vi "Retrieve and visulize data_SE.vi"(11 "Field/Temperature":i32(slide) min=0 max=36 step=1 scale=-1.1..1.0) -> (1 "slowest":dbl=-2499.957 format="%#_6p")   [LabVIEW 2016, in "Retrieve and Visualize.lvclass"]
uses:
  Retrieve and Visualize.lvclass
  typedefs/IV Setup--Cluster.ctl
  typedefs/Choose Data--enum.ctl
  <userlib>/LevyLab/LV to ITX/Data/Typedefs/File Type--enum.ctl
  <userlib>/LevyLab/Graph Utilities/graph_utilities.lvclass
  <userlib>/LevyLab/Levylab Instruments/SMOs/Configuration/Configuration.lvclass
  typedefs/INI--Cluster.ctl
  <vilib>/Utility/sysdir.llb/System Directory Type.ctl
  <userlib>/LevyLab/Graph Utilities/graph_utilities.lvclass/graph_utilities.ctl
  Retrieve and Visualize.lvclass/Retrieve and Visualize.ctl
  <userlib>/_OpenG.lib/file/file.llb/File Exists - Scalar__ogtk.vi
  <vilib>/Analysis/NI_AAL_SigProc.lvlib
  <userlib>/LevyLab/XY Utilities/xy_utilities.lvlib
  <userlib>/LevyLab/XY Utilities/subVIs/Interpolate (single).vi
  <userlib>/LevyLab/XY Utilities/Typedefs/Interpolation Configuration--cluster.ctl
  <userlib>/LevyLab/LV to ITX/Data.ITX/Data.ITX.lvclass
  <userlib>/LevyLab/LV to ITX/Data/Data.lvclass
panel:
  in  "Export ITX Name":string="B2"
  in  "Export What?":T1(ring)
  in  "Export ITX":bool
  in  "Export ITX Path":path=path "C:/"
  out "Status":string="Exit"
  out "Slow":dbl=88828.125
  out "Fast":dbl=-0.009836065573770498
  in  "OK":bool
  in  "Open DAT Path":path=path "C:/"
  in  "side points 4T":i32=8
  in  "side points 2T":i32=12
  in  "Fit Points":dbl=12.0
  in  "SG Filter?":bool=TRUE
  in  "Visualize Button":bool
  in  "Tab Control":T2(tab)=enum."Intensity Graphs"
  out "Comments":string
  in  "Check Files Button":bool
  in  "Generate Button":bool
  in  "Additional comments":string
  in  "Field Period":i32=1
  in  "# of fields/Temperatures":i32=1
  in  "Path":path=path "C:/"
  in  "DAT folder":path=path "C:/"
  in  "IV file name":string="Name.dat"
  in  "IV setup":T3={"# Vslow"=11, "# Vfast"=251, "#IV Curves at each gate"=1, "B/T offset"=0, "Discard first # curves"=0, "Manual offset"=0}
  in  "Scan names":string[](array[string])=["appliedVsg", "appliedField", "appliedField"]
  in  "Portion of data":cluster{dbl, dbl}(slide)={1.0, 0.0} scale=0.0..1.0
  in  "Decimate point":dbl=10.0 format="%#_1f"
  in  "Extract paramaters from comments?":bool=TRUE
  in  "index":T4={"A"=7, "B"=6, "C"=3, "D"=6, "E"=3, "N1"=2, "N2"=2, "N3"=3, "N4"=4, "A 1"=8, "A 2"=10, "C 1"=5, "C 2"=1, "E 2"=4}
  in  "T/B third axis":bool
  in  "File Type":T5
  out "IV":cluster{dbl[], dbl[]}[](graph)
  out "dI/dV":cluster{dbl[], dbl[]}[](graph)
  out "dI/dV 2T":cluster{dbl[], dbl[]}[](graph)
  out "IV 2T":cluster{dbl[], dbl[]}[](graph)
  out "dV/dI":cluster{dbl[], dbl[]}[](graph)
  out "dV/dI 2T":cluster{dbl[], dbl[]}[](graph)
  out "IV slow 2T":cluster{dbl[], dbl[]}[](graph)
  out "dI/dV slow 2T":cluster{dbl[], dbl[]}[](graph)
  out "IV slow 4T":cluster{dbl[], dbl[]}[](graph)
  out "dI/dV slow 4T":cluster{dbl[], dbl[]}[](graph)
  out "IV vary 3rd 2T":cluster{dbl[], dbl[]}[](graph)
  out "dI/dV vary 3rd 2T":cluster{dbl[], dbl[]}[](graph)
  out "IV vary 3rd 4T":cluster{dbl[], dbl[]}[](graph)
  out "dI/dV vary 3rd 4T":cluster{dbl[], dbl[]}[](graph)
  in  "fake point 1":dbl format="%#_6p"
  in  "Log scale? 1":bool
  in  "e^2/h? 1":bool=TRUE
  in  "derivative bin size 1":dbl=12.0
  in  "derivative bin size 2":dbl=12.0
  in  "e^2/h? 2":bool=TRUE
  in  "Log scale? 2":bool
  in  "fake point 2":dbl format="%#_6p"
  in  "Intensity 1":T6=enum."G-4T"
  out "Intensity Graph 1":dbl[][](graph)
  out "Intensity Graph 2":dbl[][](graph)
  out "H Cut 1":cluster{dbl[], dbl[]}[](graph)
  out "V Cut 1":cluster{dbl[], dbl[]}[](graph)
  out "H Cut 2":cluster{dbl[], dbl[]}[](graph)
  out "V Cut 2":cluster{dbl[], dbl[]}[](graph)
  in  "Intensity 2":T6=enum."dGdVsg-4T"
  in  "X Offset 1":dbl format="%#_6p"
  in  "X Offset 2":dbl format="%#_6p"
  out "x3D Intensity Graph 11":dbl[][](graph)
  out "x3D Intensity Graph 10":dbl[][](graph)
  out "x3D Intensity Graph 9":dbl[][](graph)
  out "x3D Transconductance 2":dbl[][](graph)
  out "bottom loop":dbl[](graph)
  out "xalpha top loop":dbl[](graph)
  out "xalpha Top loop Intensity Graph":dbl[][](graph)
  out "xalpha Vsd vs Vsg":cluster{dbl[], dbl[]}(graph)
  in  "xalpha threshold 2":dbl format="%0.2f"
  in  "xalpha width 2":i32=3 min=3
  out "xalpha Y line cut 9":cluster{dbl[], dbl[]}[](graph)
  out "xalpha Vsg?":dbl[](array[numeric])
  out "xalpha vertical peak diff":dbl[](array[numeric])
  in  "xalpha threshold":dbl format="%0.2f"
  in  "xalpha width":i32=3 min=3
  in  "xalpha derivative bin size":dbl=10.0
  out "Cursor Graph":cluster{dbl[], dbl[]}(graph)
  # "I+"
  # "V+"
  # "Vsg1"
  # "Vsgw"
  # "Vsg2"
  # "V-"
  # "I-"
  # "Input"
  # "Process Parameters"
  # "Vfast"
  # "Vslow"
  # "Vslowest"
  # "Output"
  # "Used??"
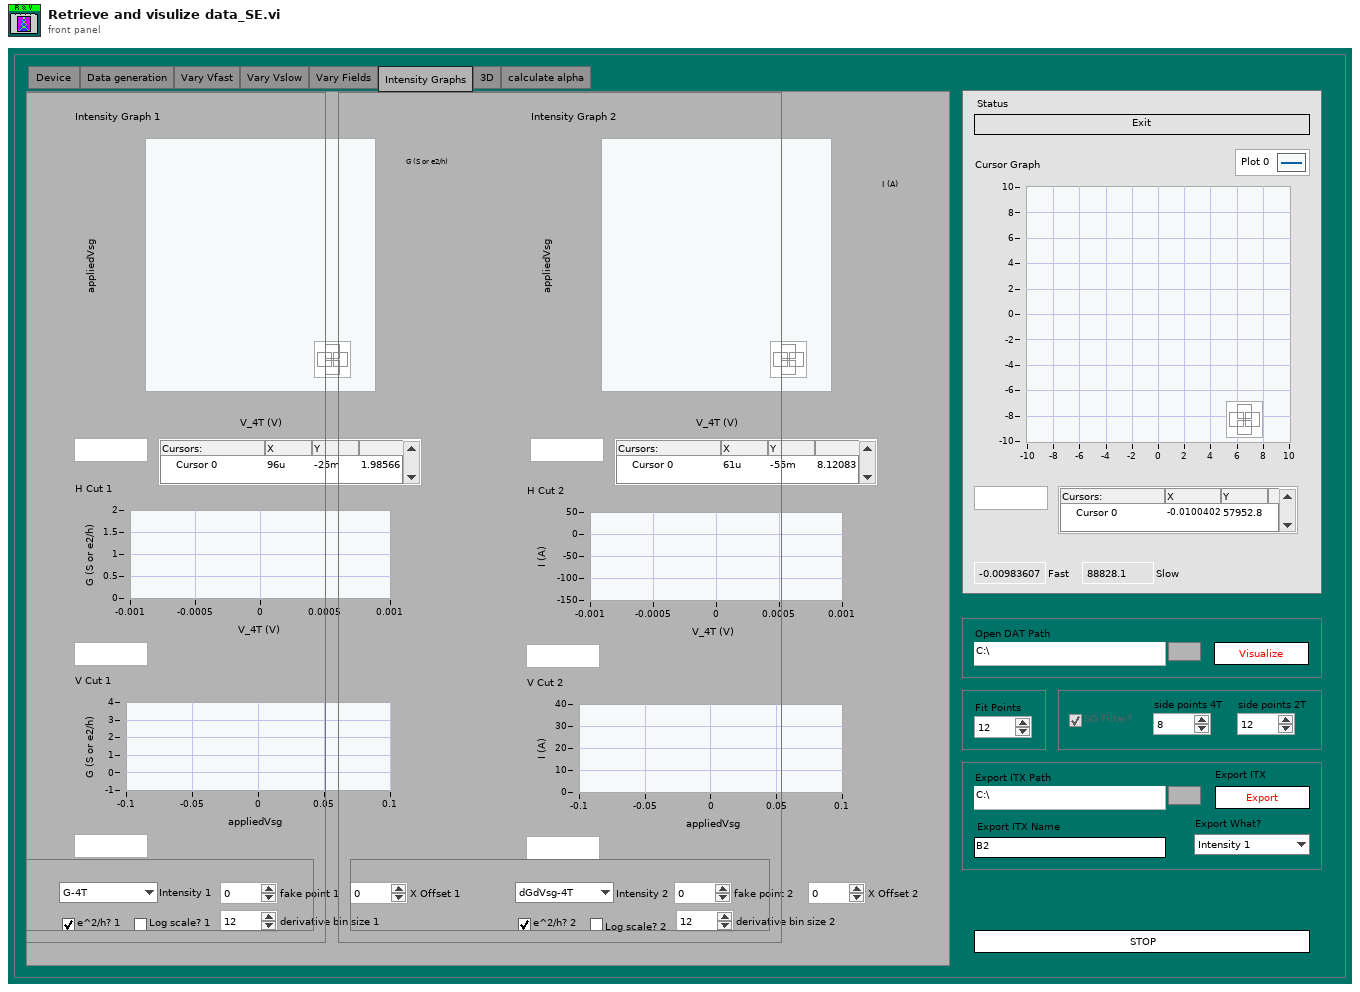
[diagram p1: front panel]
types:
  T1 = enum16{"Intensity 1", "H Cut 1", "V Cut 1", "Intensity 2", "H Cut 2", "V Cut 2"}
  T2 = enum32{"Device ", "Data generation", "Vary Vfast", "Vary Vslow", "Vary Fields", "Intensity Graphs", "3D", "calculate alpha"}
  T3 = typedef "Retrieve and Visualize.lvclass/IV Setup--Cluster.ctl" = cluster{"# Vslow":i32, "# Vfast":i32, "#IV Curves at each gate":i32, "B/T offset":i32, "Discard first # curves":i32, "Manual offset":i32}
  T4 = cluster{"A":i32, "B":i32, "C":i32, "D":i32, "E":i32, "N1":i32, "N2":i32, "N3":i32, "N4":i32, "A 1":i32, "A 2":i32, "C 1":i32, "C 2":i32, "E 2":i32}
  T5 = typedef "Data.lvclass/File Type--enum.ctl" = enum16{"DAT", "ITX", "TDMS", "VI"}
  T6 = typedef "Retrieve and Visualize.lvclass/Choose Data--enum.ctl" = enum16{"IV-4T", "IV-2T", "R-4T", "G-4T", "R-2T", "G-2T", "dGdVsg-4T"}
  T7 = enum32{"Device ", "Data generation", "Vary Vfast", "Vary Vslow", "Vary Fields", "Intensity Graphs", "3D (disabled)", "calculate alpha (disabled)"}
  T8 = cluster{"IV-4T":refnum<data-value>, "G-2T":refnum<data-value>, "R-2T":refnum<data-value>, "G-4T":refnum<data-value>, "R-4T":refnum<data-value>, "IV-2T":refnum<data-value>, "Vfast":dbl[][], "Vslow":dbl[], "Vslowest":dbl[], "Scan Names":string[]}
  T9 = typedef "xy_utilities.lvlib/Interpolation Configuration--cluster.ctl" = cluster{"X Low":dbl, "X High":dbl, "X Step":dbl, "Fake Point":dbl}
  T10 = typedef "LVOffsetAndMultiplierTypeDef.ctl" = cluster{"Offset":dbl, "Multiplier":dbl}
  T11 = enum32{"Invalid", "Standard", "Closed", "Hidden", "Minimized", "Maximized"}
  T12 = enum32{"invalid app kind", "Development System", "Run Time System", "Student Edition", "Embedded LabVIEW", "Evaluation", "Custom"}
  T13 = typedef "Retrieve and Visualize.lvclass/INI--Cluster.ctl" = cluster{"Open DAT Path":path, "Export ITX Path":path, "Export ITX Name":string, "Intensity 1":T6, "X Offset 1":dbl, "derivative bin size 1":dbl, "e^2/h? 1":bool, "Log scale? 1":bool, "fake point 1":dbl, "Intensity 2":T6, "X Offset 2":dbl, "derivative bin size 2":dbl, "e^2/h? 2":bool, "Log scale? 2":bool, "fake point 2":dbl}
  T14 = cluster{"Core":cluster{"Current VI Reference":refnum<vi>, "Close Panel on Exit?":bool}, "Retrieve and Visualize":refnum<class "Retrieve and Visualize.lvclass">, "Configuration":refnum<class "Configuration.lvclass">, "INI":T13, "DVR":cluster{"IV-4T":refnum<data-value>, "IV-2T":refnum<data-value>, "G-4T":refnum<data-value>, "R-4T":refnum<data-value>, "G-2T":refnum<data-value>, "R-2T":refnum<data-value>}, "Graph":cluster{"Intensity 1":refnum<class "graph_utilities.lvclass">, "V 1":refnum<class "graph_utilities.lvclass">, "H 1":refnum<class "graph_utilities.lvclass">, "Intensity 2":refnum<class "graph_utilities.lvclass">, "V 2":refnum<class "graph_utilities.lvclass">, "H 2":refnum<class "graph_utilities.lvclass">}, "Vfast":dbl[][], "Vslow":dbl[], "Vslowest":dbl[], "Scan Names":string[], "Vfast Slice":dbl[], "Vslow Slice":dbl[], "Page":i32, "Row Array":i32[], "Column Array":i32[], "Row":i32, "Column":i32}
  T15 = cluster{"Intensity 1":refnum<class "graph_utilities.lvclass">, "V 1":refnum<class "graph_utilities.lvclass">, "H 1":refnum<class "graph_utilities.lvclass">, "Intensity 2":refnum<class "graph_utilities.lvclass">, "V 2":refnum<class "graph_utilities.lvclass">, "H 2":refnum<class "graph_utilities.lvclass">}
  T16 = cluster{"IV-4T":refnum<data-value>, "IV-2T":refnum<data-value>, "G-4T":refnum<data-value>, "R-4T":refnum<data-value>, "G-2T":refnum<data-value>, "R-2T":refnum<data-value>}
  T17 = cluster{"Current VI Reference":refnum<vi>, "Close Panel on Exit?":bool}
  T18 = typedef "System Directory Type.ctl" = i32
  T19 = typedef "LVPointDoubleTypeDef.ctl" = cluster{"X":dbl, "Y":dbl}
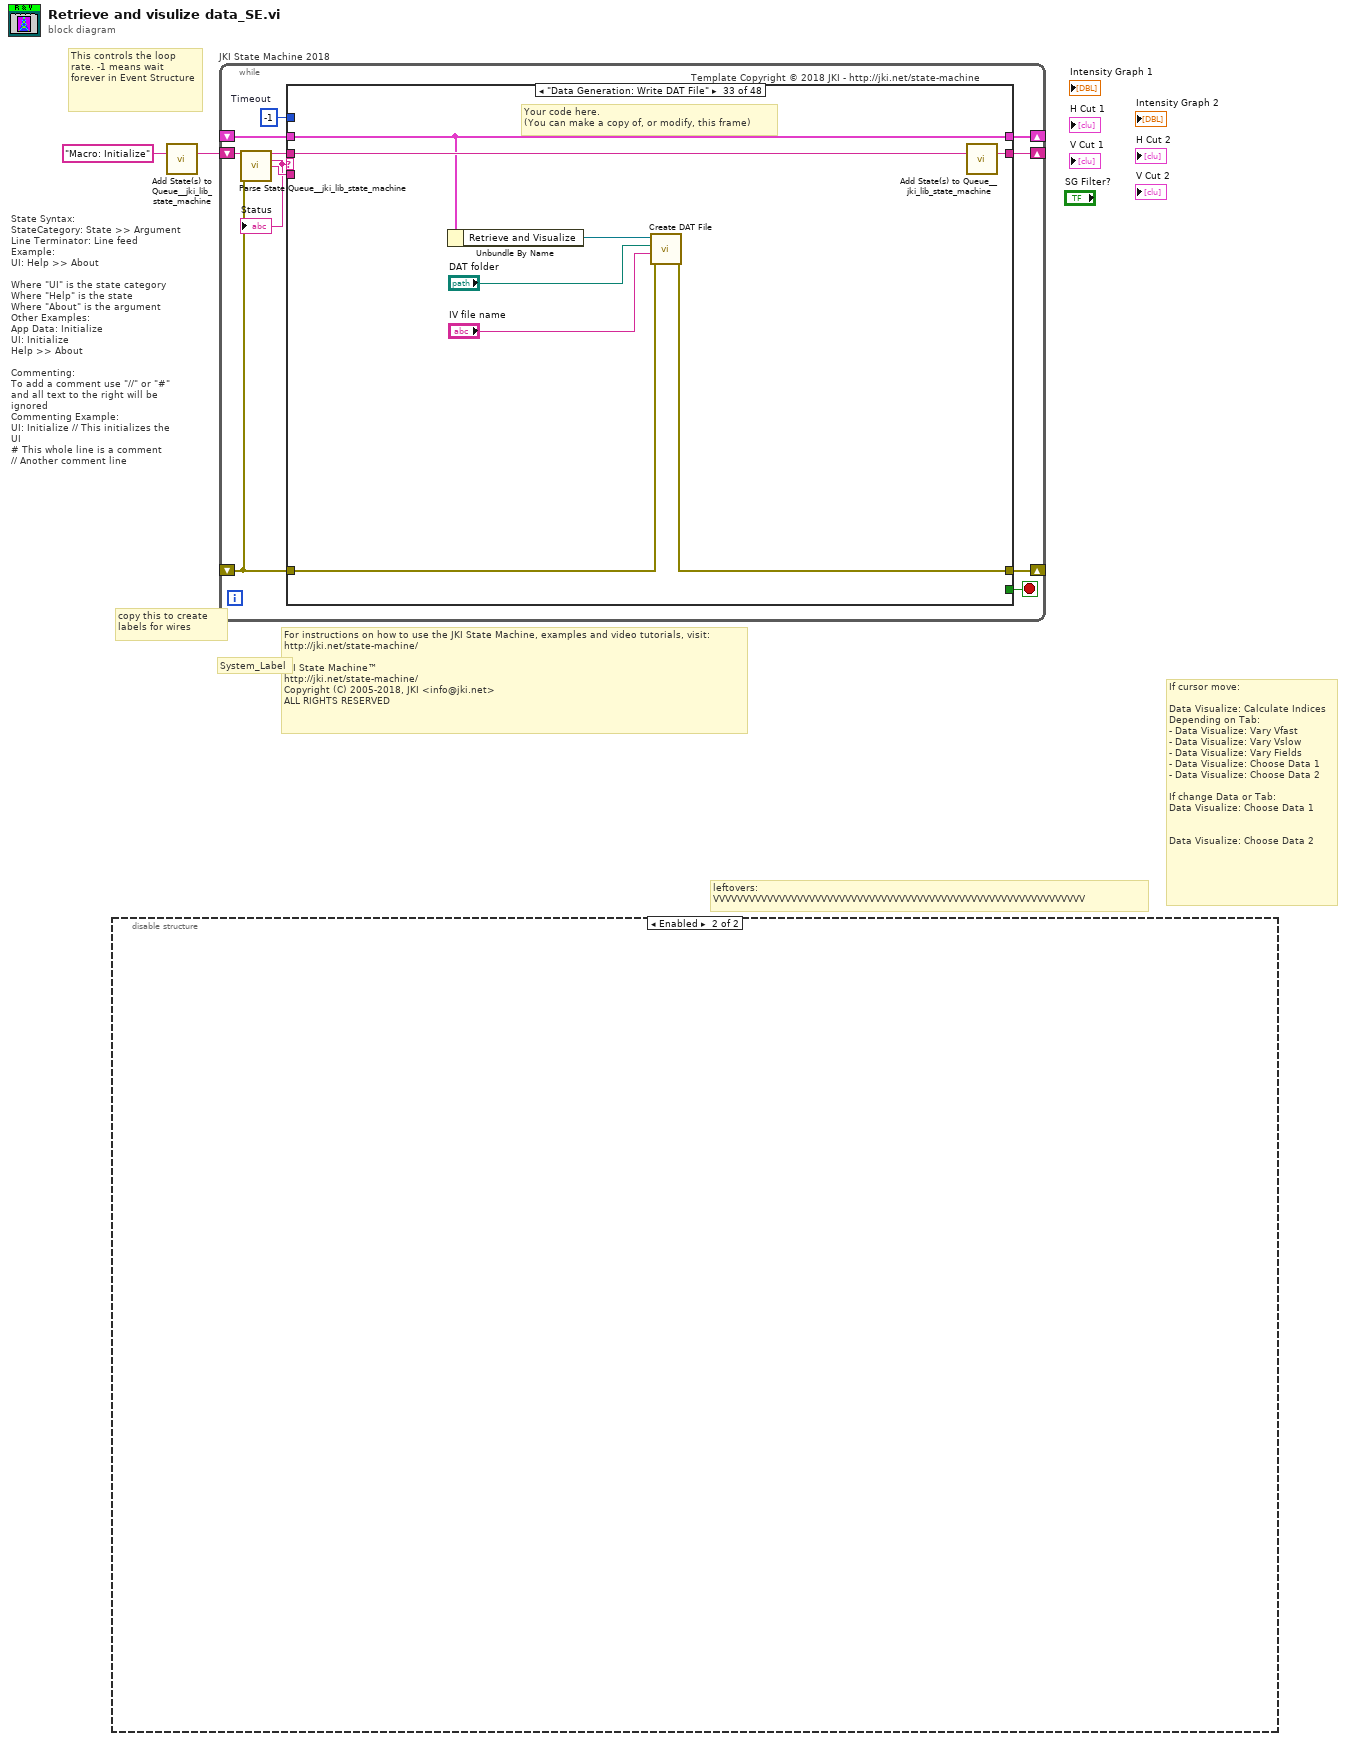
[diagram p0: block diagram]
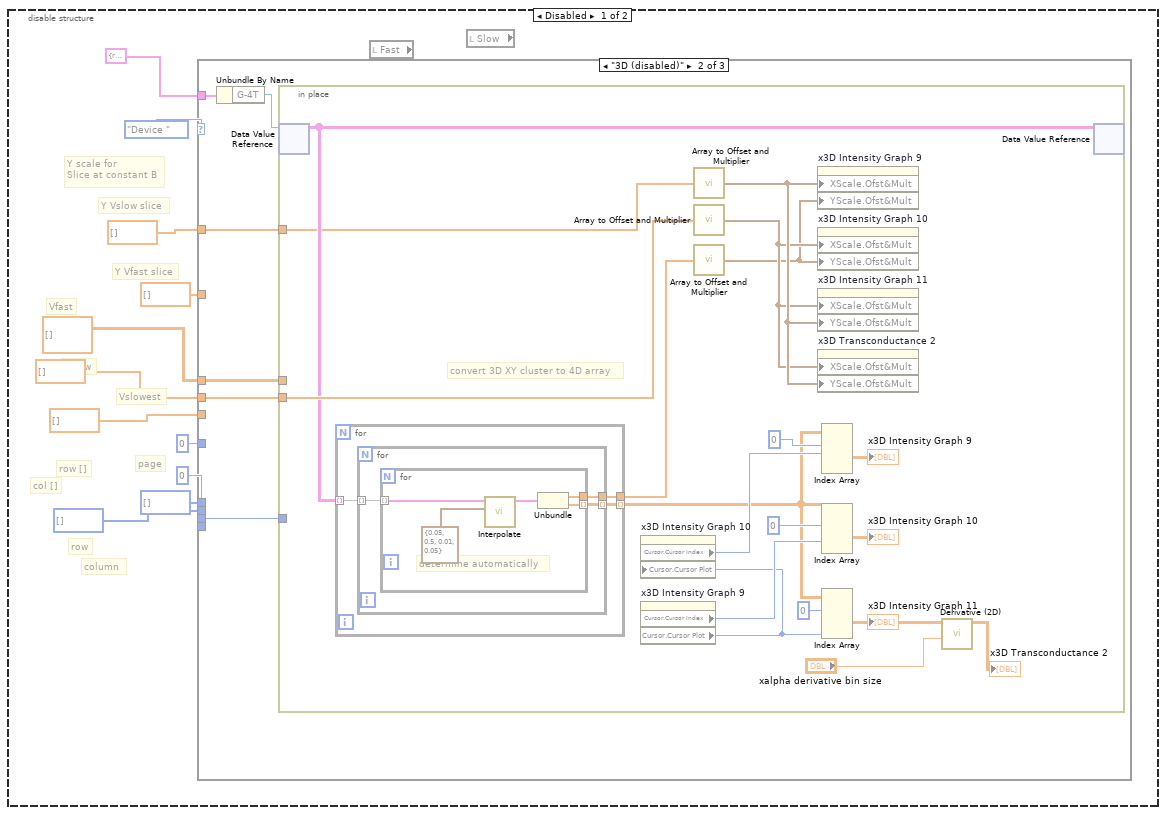
[diagram p2: hidden frame]
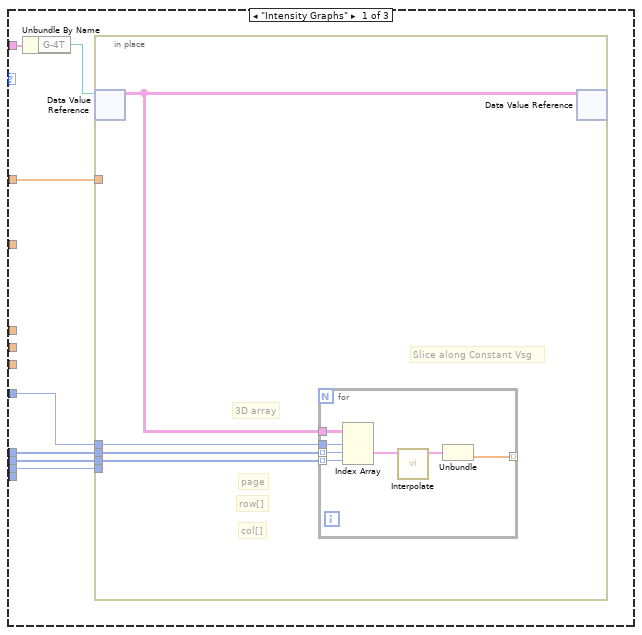
[diagram p3: hidden frame]
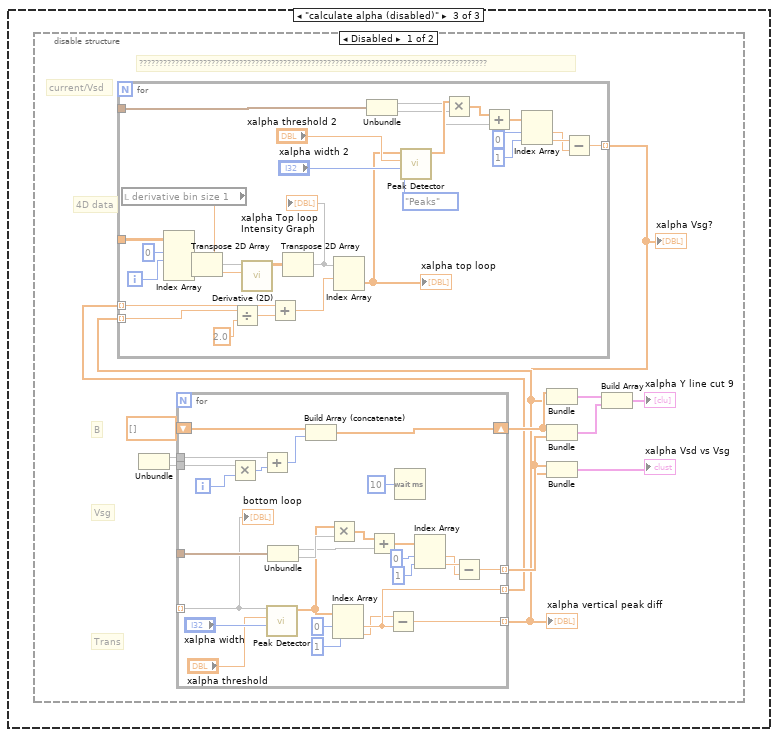
[diagram p4: hidden frame]
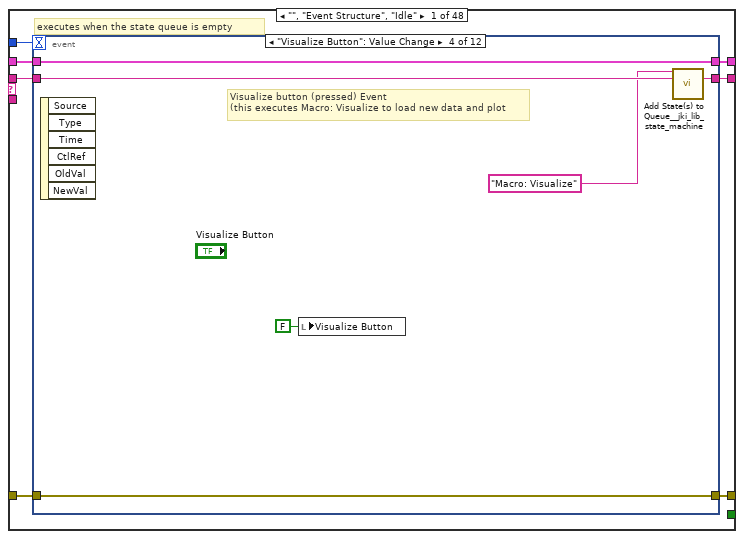
[diagram p6: hidden frame]
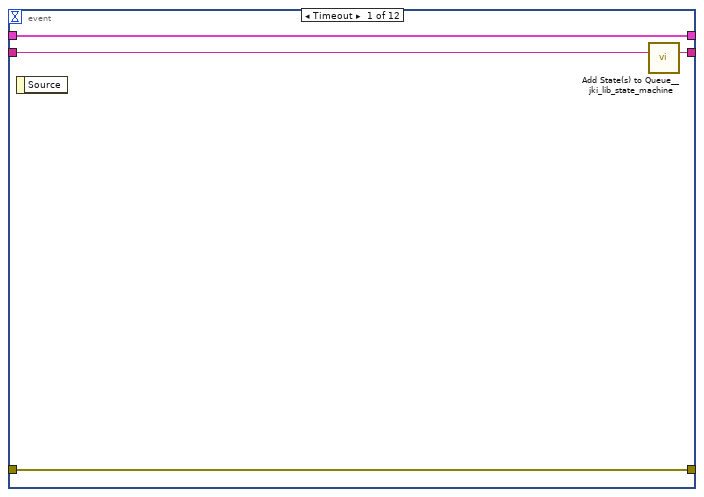
[diagram p7: hidden frame]
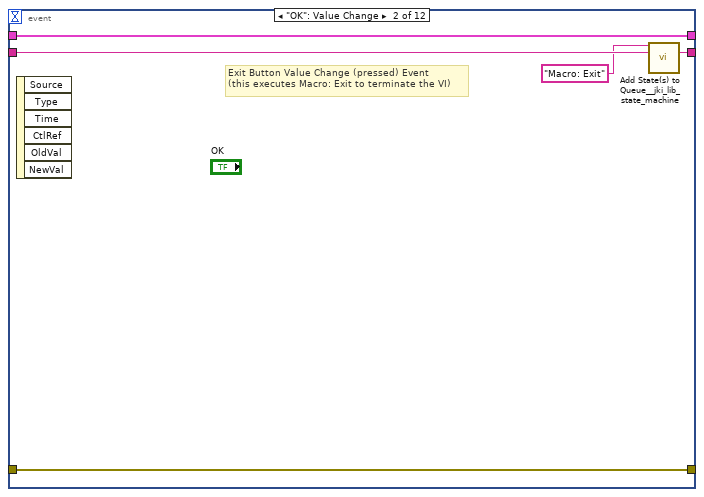
[diagram p8: hidden frame]
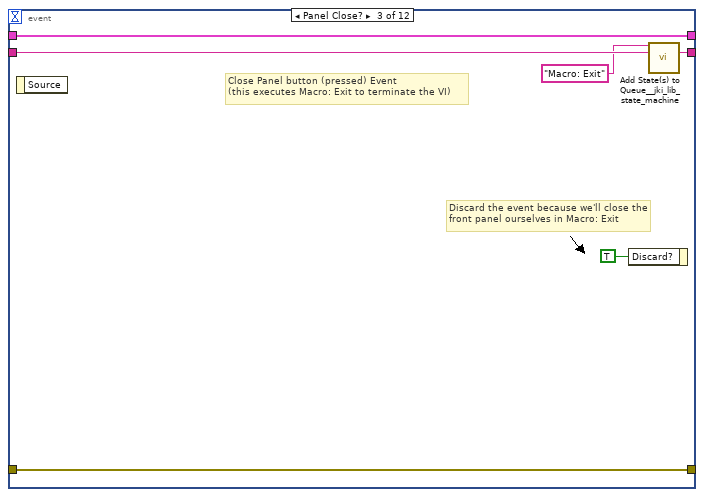
[diagram p9: hidden frame]
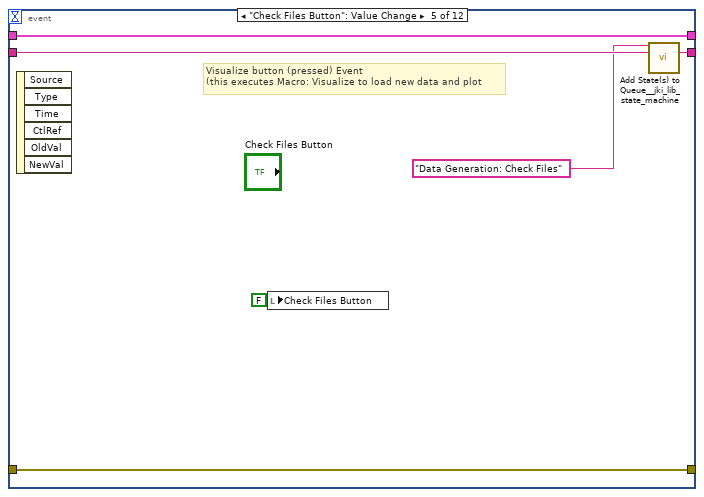
[diagram p10: hidden frame]
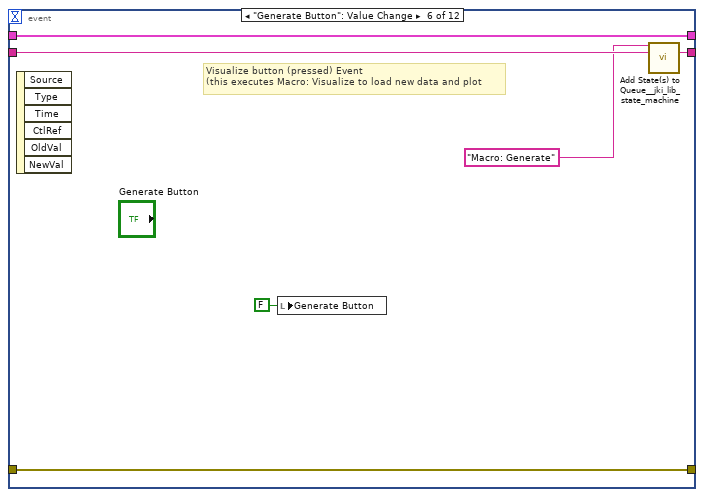
[diagram p11: hidden frame]
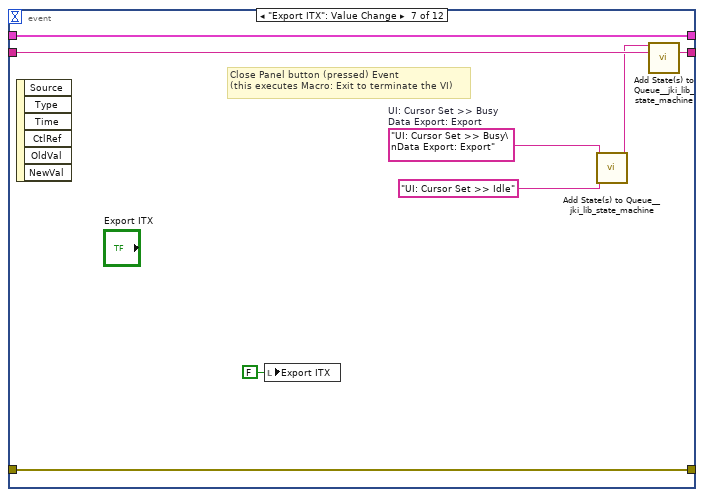
[diagram p12: hidden frame]
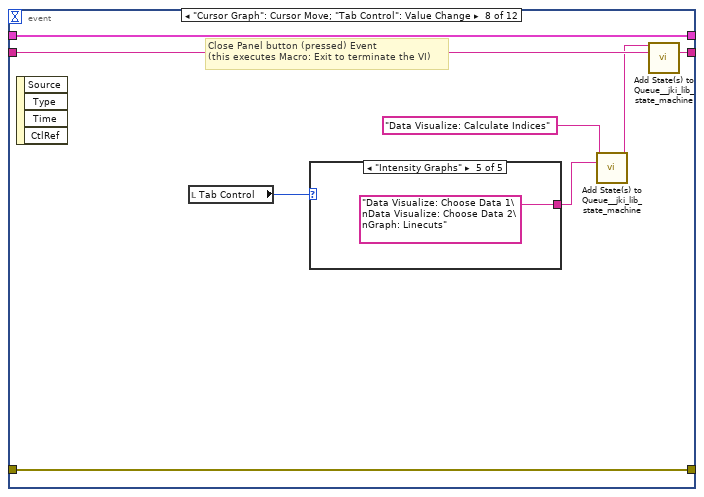
[diagram p13: hidden frame]
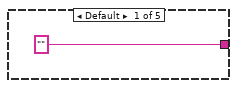
[diagram p14: hidden frame]
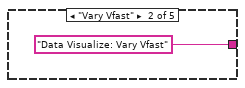
[diagram p15: hidden frame]
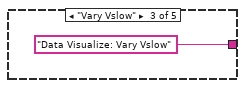
[diagram p16: hidden frame]
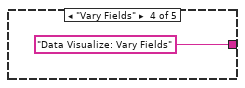
[diagram p17: hidden frame]
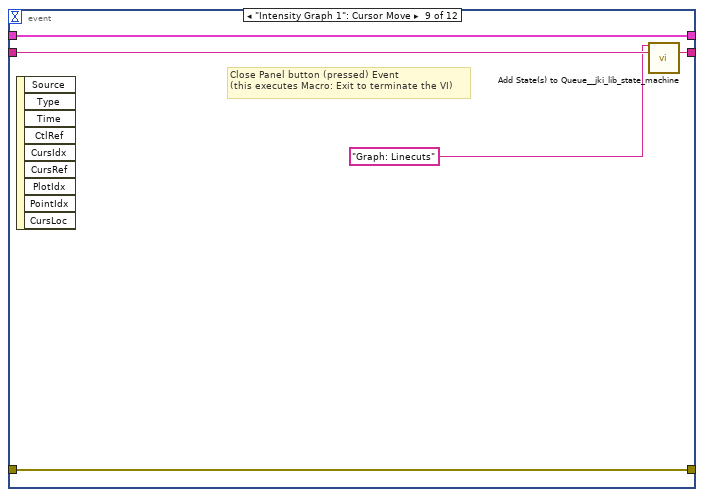
[diagram p18: hidden frame]
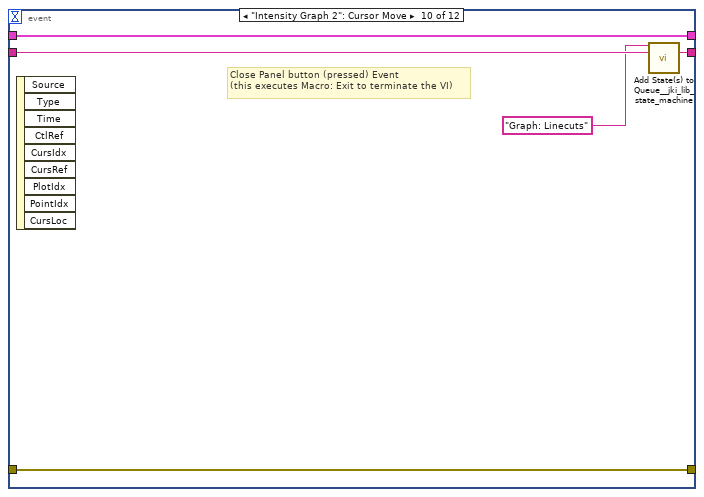
[diagram p19: hidden frame]
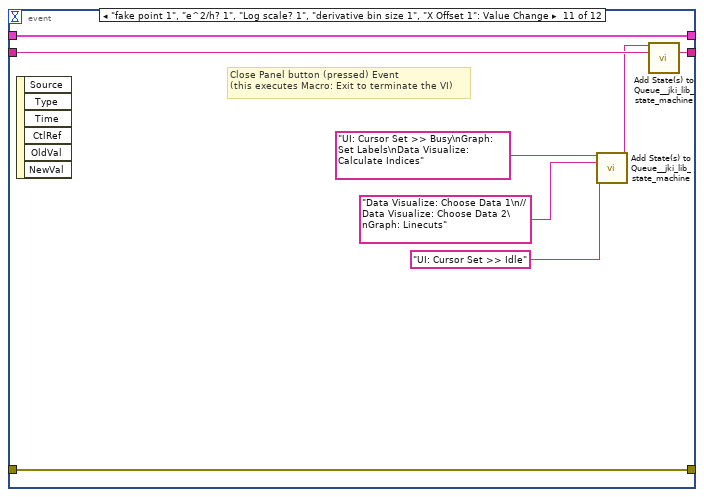
[diagram p20: hidden frame]
diagram:
  # "If cursor move:\n\nData Visualize: Calculate Indices\nDepending on Tab:\n- Data Visualize: Vary Vfast\n- Data Visualize: Vary Vslow\n- Data Visualize: Vary Fields\n- Data Visualize: Choose Data 1\n- Data Visualize: Choose Data 2\n\nIf change Data or Tab:\nData Visualize: Choose Data 1\n\n\nData Visualize: Choose Data 2"
  # "leftovers:\nVVVVVVVVVVVVVVVVVVVVVVVVVVVVVVVVVVVVVVVVVVVVVVVVVVVVVVVVVVVVVV"
  # "For instructions on how to use the JKI State Machine, examples and video tutorials, visit:\nhttp://jki.net/state-machine/\n\nJKI State Machine™\nhttp://jki.net/state-machine/\nCopyright (C) 2005-2018, JKI <info@jki.net>\nALL RIGHTS RESERVED"
  # "State Syntax:\nStateCategory: State >> Argument\nLine Terminator: Line feed\nExample:\nUI: Help >> About\n\nWhere \"UI\" is the state category\nWhere \"Help\" is the state\nWhere \"About\" is the argument\nOther Examples:\nApp Data: Initialize\nUI: Initialize\nHelp >> About\n\nCommenting:\nTo add a comment use \"//\" or \"#\" and all text to the right will be ignored\nCommenting Example:\nUI: Initialize // This initializes the UI\n# This whole line is a comment\n// Another comment line"
  # "copy this to create labels for wires"
  # "This controls the loop rate. -1 means wait forever in Event Structure"
  # "System_Label"
  n1 = disable-structure shown="Enabled" {
    frame Disabled {
      # "column"
      # "Y Vfast slice"
      # "Y Vslow slice"
      # "Y scale for \nSlice at constant B"
      # "row"
      # "col []"
      # "row []"
      # "page"
      # "Vslowest"
      # "Vslow"
      # "Vfast"
      n2 = case shown="\"3D (disabled)\"" T7."Device " ("Tab Control") {
        tunnel: 0 ("Field/Temperature") -> [w20 _ _]
        tunnel: 0 ("Row") -> [w21 w38 _]
        tunnel: dbl[][] [] ("Vfast") -> [_ w36 _]
        tunnel: dbl[] [] ("Vslow") -> [_ w37 _]
        tunnel: dbl[] [] ("Vslowest") -> [_ _ _]
        tunnel: i32[] [] ("Row Array") -> [w19 _ _]
        tunnel: i32[] [] ("Column Array") -> [w18 _ _]
        tunnel: T8 {"IV-4T"=refnum, "G-2T"=refnum, "R-2T"=refnum, "G-4T"=refnum, "R-4T"=refnum, "IV-2T"=refnum, "Vfast"=[], "Vslow"=[], "Vslowest"=[], "Scan Names"=[]} -> [w15 w35 _]
        tunnel: dbl[] [] ("Vfast") -> [w16 w33 _]
        tunnel: dbl[] [] -> [_ _ _]
        tunnel: 0 ("Column") -> [_ _ _]
        frame "Intensity Graphs" {
          n3 = Unbundle By Name(w15) -> ("G-4T"=w17:refnum<data-value>)
          n4 = in-place {
            in-place-border: w21 -> [_]
            in-place-border: w20 -> [w25]
            in-place-border: w19 -> [w24]
            in-place-border: w18 -> [w23]
            in-place-border: w16 -> [_]
            # "page"
            # "3D array"
            # "row[]"
            # "col[]"
            # "Slice along Constant Vsg"
            n5 = in-place-dvr #1(w17) -> (w22:cluster{dbl[], dbl[]}[][][])  [unwired: 1 out]
            n6 = for {
              tunnel: w22 -> [w32]
              tunnel: w25 -> [w31]
              tunnel: w24 -> [w28] mode=indexing
              tunnel: w23 -> [w29] mode=indexing
              tunnel: [w30] -> _ mode=indexing
              n7 = Index Array(array=w32, index (dim 0)=w31, index (dim 1)=w28, index (dim 2)=w29) -> (element=w27:cluster{dbl[], dbl[]})
              n8 = call-poly <userlib>:"Interpolate.vi"("XY-data"=w27) -> ("Interpolated XY-data out"=w26:cluster{"X-array":dbl[], "Y-array":dbl[]})  [unwired: 9 in, 1 out]
              n9 = Unbundle(w26) -> ("Y-array"=w30:dbl[])  [unwired: 1 out]
            }
            n10 = in-place-dvr #1(w22) -> ()  [unwired: 2 out]
          }
        }
        frame "3D (disabled)" {
          n11 = Unbundle By Name(w35) -> ("G-4T"=w34:refnum<data-value>)
          n12 = in-place {
            in-place-border: w38 -> [_]
            in-place-border: w37 -> [w46]
            in-place-border: w36 -> [_]
            in-place-border: w33 -> [w43]
            # "convert 3D XY cluster to 4D array"
            n13 = in-place-dvr #2(w34) -> (w44:cluster{dbl[], dbl[]}[][][])  [unwired: 1 out]
            n14 = for {
              tunnel: w44 -> [w60] mode=indexing
              tunnel: [w59] -> w49 mode=indexing
              tunnel: [w58] -> w39
              n15 = for {
                tunnel: w60 -> [w63] mode=indexing
                tunnel: [w62] -> w59 mode=indexing
                tunnel: [w61] -> w58
                n16 = for {
                  tunnel: w63 -> [w67] mode=indexing
                  tunnel: [w68] -> w62 mode=indexing
                  tunnel: [w65] -> w61
                  # "determine automatically"
                  n17 = call-poly <userlib>:"Interpolate.vi"("Configure"=T9 {"X Low"=0.05, "X High"=0.5, "X Step"=0.01, "Fake Point"=0.05}, "XY-data"=w67) -> ("Interpolated XY-data out"=w66:cluster{"X-array":dbl[], "Y-array":dbl[]})  [unwired: 8 in, 1 out]
                  n18 = Unbundle(w66) -> ("X-array"=w65:dbl[], "Y-array"=w68:dbl[])
                }
              }
            }
            n19 = property on="x3D Intensity Graph 9" class="IntGraph (strict)"() -> ("Cursor.Cursor Index"=w57:i32, "Cursor.Cursor Plot"=w40:i32)  [unwired: 2 in, 2 out]
            n20 = property on="x3D Intensity Graph 10" class="IntGraph (strict)"("Cursor.Cursor Plot"=w40) -> ("Cursor.Cursor Index"=w56:i32)  [unwired: 2 in, 2 out]
            n21 = call <userlib>:"Array to Offset and Multiplier.vi"("Array"=w43) -> ("Offset and Multiplier"=w47:T10)
            n22 = call <userlib>:"Array to Offset and Multiplier.vi"("Array"=w46) -> ("Offset and Multiplier"=w45:T10)
            n23 = call <userlib>:"Array to Offset and Multiplier.vi"("Array"=w39) -> ("Offset and Multiplier"=w42:T10)
            n24 = property on="x3D Intensity Graph 9" class="IntGraph (strict)"("XScale.Ofst&Mult"=w47, "YScale.Ofst&Mult"=w42) -> ()  [unwired: 2 in, 2 out]
            n25 = property on="x3D Intensity Graph 10" class="IntGraph (strict)"("XScale.Ofst&Mult"=w45, "YScale.Ofst&Mult"=w42) -> ()  [unwired: 2 in, 2 out]
            n26 = property on="x3D Intensity Graph 11" class="IntGraph (strict)"("XScale.Ofst&Mult"=w45, "YScale.Ofst&Mult"=w47) -> ()  [unwired: 2 in, 2 out]
            n27 = property on="x3D Transconductance 2" class="IntGraph (strict)"("XScale.Ofst&Mult"=w45, "YScale.Ofst&Mult"=w47) -> ()  [unwired: 2 in, 2 out]
            n28 = Index Array(array=w49, index (dim 0)=0 ("index (vol)"), index (dim 1)=w56) -> (element=→"x3D Intensity Graph 9":dbl[][])  [unwired: 2 in]
            n29 = Index Array(array=w49, index (dim 0)=0 ("disabled index (page) 2"), index (dim 2)=w57) -> (element=→"x3D Intensity Graph 10":dbl[][])  [unwired: 2 in]
            n30 = Index Array(array=w49, index (dim 0)=0 ("disabled index (row) 2"), index (dim 3)=w40) -> (element=w51:dbl[][])  [unwired: 2 in]
            "x3D Intensity Graph 11" <- w51
            n31 = call "Derivative (2D).vi"("derivative bin size"="xalpha derivative bin size", "Conductance"=w51) -> ("Transconductance"=→"x3D Transconductance 2":dbl[][])  [unwired: 8 in, 1 out]
            n32 = in-place-dvr #2(w44) -> ()  [unwired: 2 out]
          }
        }
        frame "calculate alpha (disabled)" {
          n33 = disable-structure shown="Disabled" {
            frame Disabled {
              # "???????????????????????????????????????????????????????????????????????????????????????"
              # "4D data"
              # "Trans"
              # "B"
              # "current/Vsd"
              # "Vsg"
              n34 = Unbundle() -> (w84:T10, "Offset"=w75, "Multiplier"=w74)
              n35 = for {
                tunnel: [w118] -> w85 mode=indexing
                tunnel: [w127] -> w71 mode=indexing
                tunnel: w75 -> [w138]
                tunnel: w74 -> [w137]
                shift-right: [w134] -> w78
                shift-left: dbl[] [] -> [w132]
                tunnel: [w131] -> w72 mode=indexing
                tunnel: [w128] -> w82
                tunnel: [w119] -> w77 mode=indexing
                i -> [w136]
                n36 = Multiply(x=w137, y=w136) -> (x*y=w135:i32)
                n37 = Add(x=w138, y=w135) -> (x+y=w133:i32)
                n38 = call <vilib>:"Peak Detector.vi"("width"="xalpha width", "threshold"="xalpha threshold", "X"=w118) -> ("Locations"=w124:dbl[])  [unwired: 4 in, 4 out]
                n39 = Unbundle(w128) -> ("Offset"=w125, "Multiplier"=w126)
                n40 = Build Array (concatenate)(w132, w133) -> (w134:dbl[])
                n41 = Multiply(x=w124, y=w126) -> (x*y=w129:dbl[])
                n42 = Index Array(array=w124, index #1=0 ("index"), index #2=1 ("index")) -> (element #1=w131:dbl, element #2=w130:dbl)
                n43 = Add(x=w129, y=w125) -> (x+y=w123:dbl[])
                n44 = Subtract(x=w130, y=w131) -> (x-y=w127:dbl)
                n45 = Wait (ms)(milliseconds to wait=u32 10) -> ()  [unwired: 1 out]
                n46 = Index Array(array=w123, index #1=0 ("index"), index #2=1 ("index")) -> (element #1=w120:dbl, element #2=w121:dbl)
                n47 = Subtract(x=w121, y=w120) -> (x-y=w119:dbl)
                "bottom loop" <- w118
              }
              "xalpha vertical peak diff" <- w71
              n48 = for {
                tunnel: [w113] -> w69
                tunnel: w71 -> [w100] mode=indexing
                tunnel: w72 -> [w103] mode=indexing
                tunnel: [w98] -> w83
                tunnel: [w94] -> w70 mode=indexing
                i -> [w111]
                n49 = local read "derivative bin size 1"() -> (w110:dbl)
                n50 = Index Array(array=w113, index (dim 0)=0 ("index (vol)"), index (dim 1)=w111) -> (element=w106)  [unwired: 2 in]
                n51 = Transpose 2D Array(2D array=w106) -> (transposed array=w105:void[][])
                n52 = Divide(x=w100, y=2.0) -> (x/y=w102:dbl)
                n53 = call "Derivative (2D).vi"("Axis Array"=w110, "Conductance"=w105) -> ("Transconductance"=w104:dbl[][])  [unwired: 8 in, 1 out]
                n54 = Add(x=w103, y=w102) -> (x+y=w101:dbl)
                n55 = Transpose 2D Array(2D array=w104) -> (transposed array=w87:dbl[][])
                "xalpha Top loop Intensity Graph" <- w87
                n56 = Index Array(array=w87, index (row)=w101) -> (element=w86:dbl[])  [unwired: 1 in]
                "xalpha top loop" <- w86
                n57 = Unbundle(w98) -> ("Offset"=w92, "Multiplier"=w93)
                n58 = call <vilib>:"Peak Detector.vi"("peaks/valleys"=enum32{"Peaks", "Valleys"}."Peaks", "width"="xalpha width 2", "threshold"="xalpha threshold 2", "X"=w86) -> ("Locations"=w96:dbl[])  [unwired: 3 in, 4 out]
                n59 = Multiply(x=w96, y=w93) -> (x*y=w97:dbl[])
                n60 = Add(x=w97, y=w92) -> (x+y=w95:dbl[])
                n61 = Index Array(array=w95, index #1=0 ("index"), index #2=1 ("index")) -> (element #1=w90:dbl, element #2=w91:dbl)
                n62 = Subtract(x=w91, y=w90) -> (x-y=w94:dbl)
              }
              "xalpha Vsg?" <- w70
              n63 = Bundle(w78, w70) -> (w79:cluster{dbl[], dbl[]})  [unwired: 1 in]
              n64 = Bundle(w78, w77) -> (w81:cluster{dbl[], dbl[]})  [unwired: 1 in]
              n65 = Bundle(w77, w70) -> (→"xalpha Vsd vs Vsg":cluster{dbl[], dbl[]})  [unwired: 1 in]
              n66 = Build Array(w79, w81) -> (→"xalpha Y line cut 9":cluster{dbl[], dbl[]}[])
            }
            frame Enabled {
            }
          }
        }
      }
      n67 = local read "Fast"() -> ()  [unwired: 1 out]
      n68 = local read "Slow"() -> ()  [unwired: 1 out]
    }
    frame Enabled {
    }
  }
  n69 = call <vilib>:"Add State(s) to Queue__jki_lib_state_machine.vi"("State(s) in (\"\")"="Macro: Initialize") -> ("States Out"=w2:string)  [unwired: 14 in]
  n70 = while "JKI State Machine 2018" {
    shift-right: [w145] -> _
    shift-left: _ -> [w144]
    shift-right: [w148] -> _
    shift-left: _ -> [w142]
    shift-right: [w147] -> _
    shift-left: w2 -> [w149]
    stop <- w146 stop-if-true
    w143 = -1  # Timeout
    # "Template Copyright © 2018 JKI - http://jki.net/state-machine"
    n71 = call <vilib>:"Parse State Queue__jki_lib_state_machine.vi"("State Queue"=w149, "Error In (no error)"=w142) -> ("Remaining States"=w151:string, "Current State"=w141:string, "Arguments"=w150:string)  [unwired: 11 in]
    "Status" <- w141
    n72 = case shown="\"Data Generation: Write DAT File\"" w141 {
      selector: w141 -> [_ _ w243 _ _ _ _ _ _ _ _ _ _ _ _ _ _ _ _ _ _ w540 _ _ _ _ _ _ _ _ _ _ _ _ _ _ _ _ _ _ _ _ _ _ _ _ _ _]
      tunnel: w151 -> [w158 w242 w247 w266 _ w276 w280 w301 w307 w325 w348 w352 w375 w392 w409 w422 w426 w436 w456 w462 w473 w544 w552 w557 w568 w572 w577 w582 w586 w601 w610 w633 w641 w645 w661 w694 w712 w728 w756 w775 w797 w809 w839 w872 w910 w960 w986 w995]
      tunnel: w150 -> [_ _ _ _ _ _ _ _ _ _ _ _ _ _ _ _ _ _ _ w457 w467 _ _ _ _ _ _ _ _ _ _ _ _ _ _ _ _ _ _ _ _ _ _ _ _ _ _ _]
      tunnel: w144 -> [w156 w239 w245 w259 w269 w274 w277 _ w302 w310 w331 w349 w373 w390 w406 w420 w423 w429 w438 w460 w469 w541 w549 w554 w565 w569 w574 w579 w583 w594 w607 w630 w637 w642 w657 w690 w699 w715 w754 w771 w786 w800 w832 w865 w908 w958 w983 w993]
      tunnel: [w155 w240 w249 w263 errorcluster {"status"=FALSE, "code"=0, "source"=""} ("error out") w273 w278 w298 w303 w318 w327 w350 w360 w379 w407 w410 w424 w431 w454 w458 w470 w542 w550 w555 w566 w570 w575 w580 w584 w599 w603 w631 w638 w643 w659 w682 w697 w726 w744 w759 w776 w807 w837 w870 w889 w940 w984 w991] -> w148
      tunnel: w142 -> [w154 w240 w248 w263 w268 w273 w278 w298 w304 w322 w328 w350 _ w385 w407 w411 w424 w432 w454 w459 w471 w542 w550 w555 w566 w570 w575 w580 w584 w599 w604 w631 w639 w643 w647 w683 _ w726 w745 w763 w777 w807 w837 w870 w887 w938 w984 w989]
      tunnel: [w157 w241 w246 w265 w271 w275 w279 w300 w306 w324 w347 w351 w374 w391 w408 w421 w425 w435 w455 w461 w472 w543 w551 w556 w567 w571 w576 w581 w585 w600 w609 w632 w640 w644 w660 w693 w711 w727 w755 w774 w796 w808 w838 w871 w909 w959 w985 w994] -> w147
      tunnel: [_ _ _ _ _ TRUE _ _ _ _ _ _ _ _ _ _ _ _ _ _ _ _ _ _ _ _ _ _ _ _ _ _ _ _ _ _ _ _ _ _ _ _ _ _ _ _ _ _] -> w146
      tunnel: [w153 w239 w245 w264 w269 w274 w277 w299 w302 w317 w331 w349 w372 w390 w406 w420 w423 w429 w438 w460 w469 w541 w549 w554 w565 w569 w574 w579 w583 w593 w606 w630 w637 w642 w656 w689 w699 w715 w753 w770 w785 w800 w832 w865 w908 w958 w983 w993] -> w145
      tunnel: w143 -> [w152 _ _ _ _ _ _ _ _ _ _ _ _ _ _ _ _ _ _ _ _ _ _ _ _ _ _ _ _ _ _ _ _ _ _ _ _ _ _ _ _ _ _ _ _ _ _ _]
      frame "", "Event Structure", "Idle" {
        # "executes when the state queue is empty"
        n73 = event shown="[3] \"Visualize Button\": Value Change" {
          selector: _ -> [_ _ _ _ _ _ _ _ _ _ _ _]
          dyn-events: _ -> [_ _ _ _ _ _ _ _ _ _ _ _]
          timeout: w152 -> [_ _ _ _ _ _ _ _ _ _ _ _]
          tunnel: w158 -> [w162 w167 w173 w179 w185 w191 w199 w207 w217 w222 w230 w238]
          tunnel: [w161 w166 w172 w178 w184 w190 w198 w206 w216 w221 w229 w237] -> w157
          tunnel: w156 -> [w159 w164 w170 w176 w182 w188 w196 w204 w214 w219 w227 w235]
          tunnel: [w160 w165 w171 w177 w183 w189 w197 w205 w215 w220 w228 w236] -> w155
          tunnel: w154 -> [w160 w165 w171 w177 w183 w189 w197 w205 w215 w220 w228 w236]
          tunnel: [w159 w164 w170 w176 w182 w188 w196 w204 w214 w219 w227 w235] -> w153
          event Timeout {
            n74 = event-data() -> ()  [unwired: 1 in, 1 out]
            n75 = call <vilib>:"Add State(s) to Queue__jki_lib_state_machine.vi"("State(s) in (\"\")"=w162) -> ("States Out"=w161:string)  [unwired: 14 in]
          }
          event "OK": Value Change {
            # "Exit Button Value Change (pressed) Event\n(this executes Macro: Exit to terminate the VI)"
            n76 = event-data() -> ()  [unwired: 1 in, 6 out]
            n77 = call <vilib>:"Add State(s) to Queue__jki_lib_state_machine.vi"("State(s) in Front (\"\")"="Macro: Exit", "State(s) in (\"\")"=w167) -> ("States Out"=w166:string)  [unwired: 13 in]
          }
          event Panel Close? {
            # "Discard the event because we'll close the front panel ourselves in Macro: Exit"
            # "Close Panel button (pressed) Event\n(this executes Macro: Exit to terminate the VI)"
            n78 = event-data() -> ()  [unwired: 1 in, 1 out]
            n79 = event-data("Discard?"=TRUE) -> ()  [unwired: 1 in, 1 out]
            n80 = call <vilib>:"Add State(s) to Queue__jki_lib_state_machine.vi"("State(s) in Front (\"\")"="Macro: Exit", "State(s) in (\"\")"=w173) -> ("States Out"=w172:string)  [unwired: 13 in]
          }
          event "Visualize Button": Value Change {
            # "Visualize button (pressed) Event\n(this executes Macro: Visualize to load new data and plot"
            n81 = event-data() -> ()  [unwired: 1 in, 6 out]
            n82 = local write "Visualize Button"(FALSE ("Visualize Button")) -> ()
            n83 = call <vilib>:"Add State(s) to Queue__jki_lib_state_machine.vi"("State(s) in Front (\"\")"="Macro: Visualize", "State(s) in (\"\")"=w179) -> ("States Out"=w178:string)  [unwired: 13 in]
          }
          event "Check Files Button": Value Change {
            # "Visualize button (pressed) Event\n(this executes Macro: Visualize to load new data and plot"
            n84 = event-data() -> ()  [unwired: 1 in, 6 out]
            n85 = local write "Check Files Button"(FALSE ("Visualize Button")) -> ()
            n86 = call <vilib>:"Add State(s) to Queue__jki_lib_state_machine.vi"("State(s) in Front (\"\")"="Data Generation: Check Files", "State(s) in (\"\")"=w185) -> ("States Out"=w184:string)  [unwired: 13 in]
          }
          event "Generate Button": Value Change {
            # "Visualize button (pressed) Event\n(this executes Macro: Visualize to load new data and plot"
            n87 = event-data() -> ()  [unwired: 1 in, 6 out]
            n88 = local write "Generate Button"(FALSE ("Generate Button")) -> ()
            n89 = call <vilib>:"Add State(s) to Queue__jki_lib_state_machine.vi"("State(s) in Front (\"\")"="Macro: Generate", "State(s) in (\"\")"=w191) -> ("States Out"=w190:string)  [unwired: 13 in]
          }
          event "Export ITX": Value Change {
            w195 = "UI: Cursor Set >> Busy\nData Export: Export"  # UI: Cursor Set >> Busy Data Export: Export
            # "Close Panel button (pressed) Event\n(this executes Macro: Exit to terminate the VI)"
            n90 = event-data() -> ()  [unwired: 1 in, 6 out]
            n91 = local write "Export ITX"(FALSE ("Export")) -> ()
            n92 = call <vilib>:"Add State(s) to Queue__jki_lib_state_machine.vi"("State(s) in Front (\"\")"=w195, "State(s) at Back (\"\")"="UI: Cursor Set >> Idle") -> ("States Out"=w194:string)  [unwired: 13 in]
            n93 = call <vilib>:"Add State(s) to Queue__jki_lib_state_machine.vi"("State(s) in Front (\"\")"=w194, "State(s) in (\"\")"=w199) -> ("States Out"=w198:string)  [unwired: 13 in]
          }
          event "Cursor Graph": Cursor Move; "Tab Control": Value Change {
            # "Close Panel button (pressed) Event\n(this executes Macro: Exit to terminate the VI)"
            n94 = event-data() -> ()  [unwired: 1 in, 4 out]
            n95 = local read "Tab Control"() -> (w203:T2)
            n96 = case shown="\"Intensity Graphs\"" w203 {
              tunnel: ["" "Data Visualize: Vary Vfast" "Data Visualize: Vary Vslow" "Data Visualize: Vary Fields" "Data Visualize: Choose Data 1\nData Visualize: Choose Data 2\nGraph: Linecuts"] -> w200
              frame Default {
              }
              frame "Vary Vfast" {
              }
              frame "Vary Vslow" {
              }
              frame "Vary Fields" {
              }
              frame "Intensity Graphs" {
              }
            }
            n97 = call <vilib>:"Add State(s) to Queue__jki_lib_state_machine.vi"("State(s) in Front (\"\")"="Data Visualize: Calculate Indices", "State(s) in (\"\")"=w200) -> ("States Out"=w201:string)  [unwired: 13 in]
            n98 = call <vilib>:"Add State(s) to Queue__jki_lib_state_machine.vi"("State(s) in Front (\"\")"=w201, "State(s) in (\"\")"=w207) -> ("States Out"=w206:string)  [unwired: 13 in]
          }
          event "Intensity Graph 1": Cursor Move {
            # "Close Panel button (pressed) Event\n(this executes Macro: Exit to terminate the VI)"
            n99 = event-data() -> ()  [unwired: 1 in, 9 out]
            n100 = call <vilib>:"Add State(s) to Queue__jki_lib_state_machine.vi"("State(s) in Front (\"\")"="Graph: Linecuts", "State(s) in (\"\")"=w217) -> ("States Out"=w216:string)  [unwired: 13 in]
          }
          event "Intensity Graph 2": Cursor Move {
            # "Close Panel button (pressed) Event\n(this executes Macro: Exit to terminate the VI)"
            n101 = event-data() -> ()  [unwired: 1 in, 9 out]
            n102 = call <vilib>:"Add State(s) to Queue__jki_lib_state_machine.vi"("State(s) in Front (\"\")"="Graph: Linecuts", "State(s) in (\"\")"=w222) -> ("States Out"=w221:string)  [unwired: 13 in]
          }
          event "fake point 1", "e^2/h? 1", "Log scale? 1", "derivative bin size 1", "X Offset 1": Value Change {
            # "Close Panel button (pressed) Event\n(this executes Macro: Exit to terminate the VI)"
            n103 = event-data() -> ()  [unwired: 1 in, 6 out]
            n104 = call <vilib>:"Add State(s) to Queue__jki_lib_state_machine.vi"("State(s) in Front (\"\")"="UI: Cursor Set >> Busy\nGraph: Set Labels\nData Visualize: Calculate Indices", "State(s) in (\"\")"="Data Visualize: Choose Data 1\n//Data Visualize: Choose Data 2\nGraph: Linecuts", "State(s) at Back (\"\")"="UI: Cursor Set >> Idle") -> ("States Out"=w225:string)  [unwired: 12 in]
            n105 = call <vilib>:"Add State(s) to Queue__jki_lib_state_machine.vi"("State(s) in Front (\"\")"=w225, "State(s) in (\"\")"=w230) -> ("States Out"=w229:string)  [unwired: 13 in]
          }
          event "fake point 2", "e^2/h? 2", "Log scale? 2", "derivative bin size 2", "X Offset 2": Value Change {
            # "Close Panel button (pressed) Event\n(this executes Macro: Exit to terminate the VI)"
            n106 = event-data() -> ()  [unwired: 1 in, 6 out]
            n107 = call <vilib>:"Add State(s) to Queue__jki_lib_state_machine.vi"("State(s) in Front (\"\")"="UI: Cursor Set >> Busy\nGraph: Set Labels\nData Visualize: Calculate Indices", "State(s) in (\"\")"="//Data Visualize: Choose Data 1\nData Visualize: Choose Data 2\nGraph: Linecuts", "State(s) at Back (\"\")"="UI: Cursor Set >> Idle") -> ("States Out"=w233:string)  [unwired: 12 in]
            n108 = call <vilib>:"Add State(s) to Queue__jki_lib_state_machine.vi"("State(s) in Front (\"\")"=w233, "State(s) in (\"\")"=w238) -> ("States Out"=w237:string)  [unwired: 13 in]
          }
        }
      }
      frame "---------- Core ----------" {
        # "Do not put any code in this frame.\n(it is a separator no-op)"
        n109 = call <vilib>:"Add State(s) to Queue__jki_lib_state_machine.vi"("State(s) in (\"\")"=w242) -> ("States Out"=w241:string)  [unwired: 14 in]
      }
      frame Default {
        w252 = 42 items=["No error", "Argument error", "Memory is full", "Out of zone", "End of file", "File already open", "Generic file I/O error", "File not found", "File permission error", "Disk is full", "Duplicate path", "Too many files open", "System feature not enabled", "Resource file not found", "Cannot add resource", "Resource not found", "Image not found", "Image memory error", "Pen does not exist", "Config type invalid", "Config token not found", "Config parse error", "Config memory error", "Bad external code format", "Bad external code offset", "External code not present", "Null window", "Destroy window error", "Null menu", "Print aborted", "Bad print record", "Print driver error", "Windows error during printing", "Memory error during printing", "Print dialog error", "Generic print error", "Invalid device refnum", "Device not found", "Device parameter error", "Device unit error", "Cannot open device", "Device call aborted", "Generic error", "Cancelled by user", "Object ID too low", "Object ID too high", "Object not in heap", "Unknown heap", "Unknown object (invalid DefProc)", "Unknown object (DefProc not in table)", "Message out of range", "Invalid (null) method", "Unknown message", "Manager call not supported", "Bad address", "Network operation in progress", "Network operation timed out", "Connection is busy", "Network attribute not supported", "Network error", "Address in use", "System out of memory", "Connection aborted", "Connection refused", "Not connected", "Already connected", "Connection closed", "Initialization error (interapplication manager)", "Bad occurrence", "Wait on unbound occurrence handler", "Occurrence queue overflow", "Datalog type conflict", "Unused", "Unrecognized type (interapplication manager)", "Memory corrupt", "Failed to make temporary DLL", "Old CIN version", "Drag socket not found", "Failed to load drop-object", "Failed to register OLE object", "Failed to release OLE object", "Format specifier type mismatch", "Unknown format specifier", "Too few format specifiers", "Too many format specifiers", "Scan failed", "Newer CIN version", "Error converting to variant", "Runtime menu error", "Password tampered", "Variant attribute not found", "Incompatible variant data type", "Event data is not available", "Event Store is not present", "Occurrence is not found", "Event Queue is not created", "Event info is not available", "Refnum passed is NULL", "Error retrieving Class GUID", "Error retrieving CoClass GUID", "Error retrieving TypeLib GUID.", "Bad built application magic bytes.", "Specific driver is different from the specific driver associated with the Logical Name.", "There is no session opened to the class driver.", "Max Error", "MAX - Error with config objects", "MAX - Error loading configuration", "MAX - Group not supported"]
        # "Current State"
        # "Do not delete, rename, or modify this frame.\n(this is used to capture unhandled states and typos)"
        # "Handle mistyped state name (developer tool)"
        n110 = Format Into String(format string="Software Exception: Unhandled State \"%s\"." ("message"), error in=w248, w243) -> (resulting string=w251:string, error out=w250:errorcluster)  [unwired: 1 in]
        n111 = call <vilib>:"Error Cluster From Error Code.vi"("show call chain? (False)"=TRUE, "error in (no error)"=w250, "error message (\"\")"=w251, "error code (0)"=w252) -> ("error out"=w249:errorcluster)  [unwired: 5 in]
        n112 = call <vilib>:"Add State(s) to Queue__jki_lib_state_machine.vi"("State(s) in (\"\")"=w247) -> ("States Out"=w246:string)  [unwired: 14 in]
      }
      frame "Initialize Core Data" {
        # "Do not delete, rename, or modify this frame.\n(this is used to determine panel behavior on exit)"
        # "originally closed?"
        # "exe?"
        # "If panel starts closed or is an EXE, then close it when we exit"
        n113 = property class="VI"() -> ("FP.State"=w256:T11)  [unwired: 2 in, 2 out]
        n114 = property class="App"() -> ("App.Kind"=w262:T12)  [unwired: 2 in, 2 out]
        n115 = control-ref of="Current VI Reference"() -> (w257:refnum<vi>)
        n116 = Equal?(x=w256, y=T11."Closed" ("Front Panel Window:State")) -> (x = y?=w254:bool)
        n117 = Equal?(x=w262, y=T12."Run Time System" ("Application:Kind")) -> (x = y?=w260:bool)
        n118 = Or(x=w254, y=w260) -> (x .or. y?=w258:bool)
        n119 = Bundle By Name(cluster=w259, "Core.Current VI Reference"=w257, "Core.Close Panel on Exit?"=w258) -> (w264:T14)
        n120 = call <vilib>:"Add State(s) to Queue__jki_lib_state_machine.vi"("State(s) in (\"\")"=w266) -> ("States Out"=w265:string)  [unwired: 14 in]
      }
      frame "Error Handler" {
        # "Unhandled Error -- Display it"
        # "Handle any errors here.\nYou can also output any states to clean-up after errors occur"
        # "Clear error"
        n121 = call <vilib>:"General Error Handler.vi"("error in (no error)"=w268) -> ()  [unwired: 10 in, 5 out]
        n122 = call <vilib>:"Add State(s) to Queue__jki_lib_state_machine.vi"("State(s) in Front (\"\")"="/* Post Error States") -> ("States Out"=w271:string)  [unwired: 14 in]
      }
      frame "Exit" {
        # "Do not put any code in this frame.\n(No errors that occur here will be handled.)"
        n123 = call <vilib>:"Add State(s) to Queue__jki_lib_state_machine.vi"("State(s) in (\"\")"=w276) -> ("States Out"=w275:string)  [unwired: 14 in]
      }
      frame "---------- Data ----------" {
        # "Do not put any code in this frame.\n(It is a separator no-op. You can make a copy of this frame to create a new Data frame)"
        n124 = call <vilib>:"Add State(s) to Queue__jki_lib_state_machine.vi"("State(s) in (\"\")"=w280) -> ("States Out"=w279:string)  [unwired: 14 in]
      }
      frame "Data: Initialize" {
        w281 = T13 {"Open DAT Path"=path "", "Export ITX Path"=path "", "Export ITX Name"="", "Intensity 1"=enum."IV-4T", "X Offset 1"=0.0, "derivative bin size 1"=0.0, "e^2/h? 1"=FALSE, "Log scale? 1"=FALSE, "fake point 1"=0.0, "Intensity 2"=enum."IV-4T", "X Offset 2"=0.0, "derivative bin size 2"=0.0, "e^2/h? 2"=FALSE, "Log scale? 2"=FALSE, "fake point 2"=0.0}  # INI
        w282 = refnum<class "Configuration.lvclass"> refnum  # Configuration
        w283 = T15 {"Intensity 1"=refnum, "V 1"=refnum, "H 1"=refnum, "Intensity 2"=refnum, "V 2"=refnum, "H 2"=refnum}  # Graph
        w284 = 0  # Column
        w289 = dbl[] []  # Vslow Slice
        w290 = dbl[] []  # Vfast Slice
        w285 = 0  # Row
        w286 = i32[] []  # Column Array
        w287 = i32[] []  # Row Array
        w288 = 0  # Page
        w291 = T16 {"IV-4T"=refnum, "IV-2T"=refnum, "G-4T"=refnum, "R-4T"=refnum, "G-2T"=refnum, "R-2T"=refnum}  # DVR
        w292 = string[] []  # Scan Names
        w293 = dbl[] []  # Vslowest
        w294 = dbl[] []  # Vslow
        w295 = dbl[][] []  # Vfast
        w296 = refnum<class "Retrieve and Visualize.lvclass"> refnum  # Retrieve and Visualize
        w297 = T17 {"Current VI Reference"=refnum, "Close Panel on Exit?"=FALSE}  # Core
        # "Initialize the shift-register data, here.\n(data names are defined by what you wire into the bundle function)"
        n125 = Bundle("Core"=w297, "Retrieve and Visualize"=w296, "Configuration"=w282, "INI"=w281, "DVR"=w291, "Graph"=w283, "Vfast"=w295, "Vslow"=w294, "Vslowest"=w293, "Scan Names"=w292, "Vfast Slice"=w290, "Vslow Slice"=w289, "Page"=w288, "Row Array"=w287, "Column Array"=w286, "Row"=w285, "Column"=w284) -> (w299:T14)  [unwired: 1 in]
        n126 = call <vilib>:"Add State(s) to Queue__jki_lib_state_machine.vi"("State(s) in (\"\")"=w301) -> ("States Out"=w300:string)  [unwired: 14 in]
      }
      frame "Data: Cleanup" {
        # "Cleanup any data and references, here.\n(this is called automatically, by the Macro: Exit)"
        n127 = Unbundle By Name(w302) -> ("Core.Current VI Reference"=w305:refnum<vi>)
        n128 = Close Reference(reference=w305, error in (no error)=w304) -> (error out=w303:errorcluster)
        n129 = call <vilib>:"Add State(s) to Queue__jki_lib_state_machine.vi"("State(s) in (\"\")"=w307) -> ("States Out"=w306:string)  [unwired: 14 in]
      }
      frame "Data: Read INI" {
        w315 = T18 3 items=["User Home"=0, "User Desktop"=1, "User Documents"=2, "User Application Data"=3, "User Preferences"=4, "User Temporary"=5, "Public Documents"=6, "Public Application Data"=7, "Public Preferences"=8, "Public Cache"=13, "System Core Libraries"=9, "System Installed Libraries"=10, "Application Files"=11, "Boot Volume Root"=12] ("system directory type")
        # "Do not put any code in this frame.\n(It is a separator no-op. You can make a copy of this frame to create a new Data frame)"
        n130 = Unbundle By Name(w310) -> ("Configuration"=w308:refnum<class "Configuration.lvclass">, "INI"=w309:T13)
        n131 = call <vilib>:"Get System Directory.vi"("system directory type"=w315) -> ("system directory"=w312:path)  [unwired: 10 in]
        n132 = Build Path(base path=w312, name or relative path="LevyLab\\Retrieve and Visualize") -> (appended path=w314:path)
        n133 = call-dynamic "Write Path.vi"("error in (no error)"=w322, "Path"=w314, "Configuration in"=w308) -> ("error out"=w321:errorcluster, "Configuration out"=w323:refnum<class "Configuration.lvclass">)  [unwired: 7 in]
        n134 = call <userlib>:"Read Configuration.vi"("INI Fomatted Cluster Type"=w309, "error in (no error)"=w321, "Configuration in"=w323) -> ("error out"=w319:errorcluster, "Configuration"=w320:variant, "Configuration out"=w316:refnum<class "Configuration.lvclass">)  [unwired: 6 in]
        n135 = Variant To Data(error in=w319, type=w309, Variant=w320) -> (data=w313:T13, error out=w318:errorcluster)
        n136 = Bundle By Name(cluster=w310, "Configuration"=w316, "INI"=w313) -> (w317:T14)
        n137 = call <vilib>:"Add State(s) to Queue__jki_lib_state_machine.vi"("State(s) in (\"\")"=w325) -> ("States Out"=w324:string)  [unwired: 14 in]
      }
      frame "Data: Write INI" {
        # "Do not put any code in this frame.\n(It is a separator no-op. You can make a copy of this frame to create a new Data frame)"
        n138 = local read "fake point 2"() -> (w332:dbl)
        n139 = local read "Open DAT Path"() -> (w346:path)
        n140 = local read "Export ITX Path"() -> (w345:path)
        n141 = local read "Export ITX Name"() -> (w344:string)
        n142 = local read "Intensity 1"() -> (w343:T6)
        n143 = local read "X Offset 1"() -> (w342:dbl)
        n144 = local read "derivative bin size 1"() -> (w341:dbl)
        n145 = local read "e^2/h? 1"() -> (w340:bool)
        n146 = local read "Log scale? 1"() -> (w339:bool)
        n147 = local read "fake point 1"() -> (w338:dbl)
        n148 = local read "Intensity 2"() -> (w337:T6)
        n149 = local read "X Offset 2"() -> (w336:dbl)
        n150 = local read "derivative bin size 2"() -> (w335:dbl)
        n151 = local read "e^2/h? 2"() -> (w334:bool)
        n152 = local read "Log scale? 2"() -> (w333:bool)
        n153 = Unbundle By Name(w331) -> ("Configuration"=w330:refnum<class "Configuration.lvclass">, "INI"=w326:T13)
        n154 = Bundle By Name(cluster=w326, "Open DAT Path"=w346, "Export ITX Path"=w345, "Export ITX Name"=w344, "Intensity 1"=w343, "X Offset 1"=w342, "derivative bin size 1"=w341, "e^2/h? 1"=w340, "Log scale? 1"=w339, "fake point 1"=w338, "Intensity 2"=w337, "X Offset 2"=w336, "derivative bin size 2"=w335, "e^2/h? 2"=w334, "Log scale? 2"=w333, "fake point 2"=w332) -> (w329:T13)
        n155 = call <userlib>:"Write Configuration.vi"("error in (no error)"=w328, "Variant"=w329, "Configuration in"=w330) -> ("error out"=w327:errorcluster)  [unwired: 7 in, 1 out]
        n156 = call <vilib>:"Add State(s) to Queue__jki_lib_state_machine.vi"("State(s) in (\"\")"=w348) -> ("States Out"=w347:string)  [unwired: 14 in]
      }
      frame "---------- Graph ----------" {
        # "Do not put any code in this frame.\n(It is a separator no-op. You can make a copy of this frame to create a new Data frame)"
        n157 = call <vilib>:"Add State(s) to Queue__jki_lib_state_machine.vi"("State(s) in (\"\")"=w352) -> ("States Out"=w351:string)  [unwired: 14 in]
      }
      frame "Graph: Initialize" {
        # "Do not put any code in this frame.\n(It is a separator no-op. You can make a copy of this frame to create a new Data frame)"
        n158 = control-ref of="Intensity Graph 1"() -> (w367:refnum<vi>)
        n159 = control-ref of="H Cut 1"() -> (w371:refnum<vi>)
        n160 = control-ref of="V Cut 1"() -> (w370:refnum<vi>)
        n161 = control-ref of="Intensity Graph 2"() -> (w353:refnum<vi>)
        n162 = control-ref of="H Cut 2"() -> (w368:refnum<vi>)
        n163 = control-ref of="V Cut 2"() -> (w369:refnum<vi>)
        n164 = call <userlib>:"Write Intensity Graph ref.vi"("Intensity Graph (Control)"=w353, "Intensity Graph"=w353) -> ("error out"=w356:errorcluster, "graph_utilities out"=w363:refnum<class "graph_utilities.lvclass">)  [unwired: 8 in]
        n165 = call <userlib>:"Write Intensity Graph ref.vi"("Intensity Graph (Control)"=w367, "Intensity Graph"=w367) -> ("error out"=w357:errorcluster, "graph_utilities out"=w366:refnum<class "graph_utilities.lvclass">)  [unwired: 8 in]
        n166 = call <userlib>:"Write XY Graph ref.vi"("XY Graph"=w368, "graph_utilities in"=w363) -> ("error out"=w355:errorcluster, "graph_utilities out"=w362:refnum<class "graph_utilities.lvclass">)  [unwired: 8 in]
        n167 = call <userlib>:"Write XY Graph ref.vi"("XY Graph"=w371, "graph_utilities in"=w366) -> ("error out"=w358:errorcluster, "graph_utilities out"=w365:refnum<class "graph_utilities.lvclass">)  [unwired: 8 in]
        n168 = call <userlib>:"Write XY Graph ref.vi"("XY Graph"=w369, "graph_utilities in"=w363) -> ("error out"=w354:errorcluster, "graph_utilities out"=w361:refnum<class "graph_utilities.lvclass">)  [unwired: 8 in]
        n169 = call <userlib>:"Write XY Graph ref.vi"("XY Graph"=w370, "graph_utilities in"=w366) -> ("error out"=w359:errorcluster, "graph_utilities out"=w364:refnum<class "graph_utilities.lvclass">)  [unwired: 8 in]
        n170 = Bundle By Name(cluster=w373, "Graph.Intensity 1"=w366, "Graph.H 1"=w365, "Graph.V 1"=w364, "Graph.Intensity 2"=w363, "Graph.H 2"=w362, "Graph.V 2"=w361) -> (w372:T14)
        n171 = Merge Errors(w357, w358, w359, w356, w355, w354) -> (w360:errorcluster)
        n172 = call <vilib>:"Add State(s) to Queue__jki_lib_state_machine.vi"("State(s) in (\"\")"=w375) -> ("States Out"=w374:string)  [unwired: 14 in]
      }
      frame "Graph: Set Y" {
        # "Do not put any code in this frame.\n(It is a separator no-op. You can make a copy of this frame to create a new Data frame)"
        n173 = Unbundle By Name(w390) -> ("Graph.Intensity 1"=w388:refnum<class "graph_utilities.lvclass">, "Graph.Intensity 2"=w387:refnum<class "graph_utilities.lvclass">, "Scan Names"=w386:string[], "Vfast Slice"=w377:dbl[], "Vslow Slice"=w376:dbl[])
        n174 = Index Array(array=w386) -> (element #1=w389:string, element #2=w378:string)  [unwired: 2 in]
        n175 = call <userlib>:"Set Intensity Graph Y Label.vi"("error in (no error)"=w385, "Y Label"=w389, "graph_utilities in"=w388) -> ("error out"=w383:errorcluster, "graph_utilities out"=w382:refnum<class "graph_utilities.lvclass">)  [unwired: 7 in]
        n176 = call <userlib>:"Set Intensity Graph Y Scale Array.vi"("error in (no error)"=w383, "Y Scale"=w377, "graph_utilities in"=w382) -> ("error out"=w381:errorcluster)  [unwired: 7 in, 1 out]
        n177 = call <userlib>:"Set Intensity Graph Y Label.vi"("error in (no error)"=w381, "Y Label"=w389, "graph_utilities in"=w387) -> ("error out"=w380:errorcluster, "graph_utilities out"=w384:refnum<class "graph_utilities.lvclass">)  [unwired: 7 in]
        n178 = call <userlib>:"Set Intensity Graph Y Scale Array.vi"("error in (no error)"=w380, "Y Scale"=w377, "graph_utilities in"=w384) -> ("error out"=w379:errorcluster)  [unwired: 7 in, 1 out]
        n179 = flat-sequence {
          tunnel: w378 -> [_]
          tunnel: w376 -> [_]
          frame #0 {
          }
        }
        n180 = call <vilib>:"Add State(s) to Queue__jki_lib_state_machine.vi"("State(s) in (\"\")"=w392) -> ("States Out"=w391:string)  [unwired: 14 in]
      }
      frame "Graph: Set Labels" {
        w393 = string[][] [["IV", "V_4T (V)", "I (A)"], ["IV-2T", "V_2T (V)", "I (A)"], ["d/dx(IV) R", "I (A)", "R (ohms or h/e2)"], ["d/dy(IV) G", "V_4T (V)", "G (S or e2/h)"], ["d/dx(IV-2T) R", "I (A)", "R (ohms or h/e2)"], ["d/dy(IV-2T) G", "V_2T (V)", "G (S or e2/h)"], ["d2/dy2(IV) dG/dVsg", "V_4T (V)", "dG/dVsg (e2/h/V or e2/h/meV)"], ["d2/dx2(IV) dR/dI", "I (A)", "dR/dI (h/e2/A)"]]
        # "Z scale"
        # "x scale"
        # "data"
        # "Z Scale & Label"
        # "X Scale & Label"
        # "Data Choice"
        # "Do not put any code in this frame.\n(It is a separator no-op. You can make a copy of this frame to create a new Data frame)"
        n181 = Unbundle By Name(w406) -> ("Graph.Intensity 1"=w405:refnum<class "graph_utilities.lvclass">, "Graph.Intensity 2"=w402:refnum<class "graph_utilities.lvclass">)
        n182 = Index Array(array=w393, index (row)="Intensity 1") -> (element=w401:string[])  [unwired: 1 in]
        n183 = Index Array(array=w393, index (row)="Intensity 2") -> (element=w400:string[])  [unwired: 1 in]
        n184 = Index Array(array=w401) -> (element #2=w397:string, element #3=w396:string)  [unwired: 3 in, 1 out]
        n185 = Index Array(array=w400) -> (element #2=w395:string, element #3=w394:string)  [unwired: 3 in, 1 out]
        n186 = call <userlib>:"Set Intensity Graph X Label.vi"("X Label"=w397, "graph_utilities in"=w405) -> ("graph_utilities out"=w404:refnum<class "graph_utilities.lvclass">)  [unwired: 8 in, 1 out]
        n187 = call <userlib>:"Set Intensity Graph Z Label.vi"("Z Label"=w396, "graph_utilities in"=w404) -> ()  [unwired: 8 in, 2 out]
        n188 = call <userlib>:"Set Intensity Graph X Label.vi"("X Label"=w395, "graph_utilities in"=w402) -> ("graph_utilities out"=w403:refnum<class "graph_utilities.lvclass">)  [unwired: 8 in, 1 out]
        n189 = call <userlib>:"Set Intensity Graph Z Label.vi"("Z Label"=w394, "graph_utilities in"=w403) -> ()  [unwired: 8 in, 2 out]
        n190 = call <vilib>:"Add State(s) to Queue__jki_lib_state_machine.vi"("State(s) in (\"\")"=w409) -> ("States Out"=w408:string)  [unwired: 14 in]
      }
      frame "Graph: Linecuts" {
        # "Do not put any code in this frame.\n(It is a separator no-op. You can make a copy of this frame to create a new Data frame)"
        n191 = Unbundle By Name(w420) -> ("Graph.V 1"=w419:refnum<class "graph_utilities.lvclass">, "Graph.H 1"=w416:refnum<class "graph_utilities.lvclass">, "Graph.V 2"=w417:refnum<class "graph_utilities.lvclass">, "Graph.H 2"=w418:refnum<class "graph_utilities.lvclass">)  [unwired: 2 out]
        n192 = call <userlib>:"Intensity Graph Linecut (Vertical).vi"("error in (no error)"=w411, "graph_utilities in"=w419) -> ("error out"=w415:errorcluster)  [unwired: 8 in, 1 out]
        n193 = call <userlib>:"Intensity Graph Linecut (Horizontal).vi"("error in (no error)"=w411, "graph_utilities in"=w416) -> ("error out"=w414:errorcluster)  [unwired: 8 in, 1 out]
        n194 = call <userlib>:"Intensity Graph Linecut (Vertical).vi"("error in (no error)"=w411, "graph_utilities in"=w417) -> ("error out"=w413:errorcluster)  [unwired: 8 in, 1 out]
        n195 = call <userlib>:"Intensity Graph Linecut (Horizontal).vi"("error in (no error)"=w411, "graph_utilities in"=w418) -> ("error out"=w412:errorcluster)  [unwired: 8 in, 1 out]
        n196 = Merge Errors(w415, w414, w413, w412) -> (w410:errorcluster)
        n197 = call <vilib>:"Add State(s) to Queue__jki_lib_state_machine.vi"("State(s) in (\"\")"=w422) -> ("States Out"=w421:string)  [unwired: 14 in]
      }
      frame "---------- UI ----------" {
        # "Do not put any code in this frame.\n(It is a separator no-op. You can make a copy of this frame to create a new UI frame)"
        n198 = call <vilib>:"Add State(s) to Queue__jki_lib_state_machine.vi"("State(s) in (\"\")"=w426) -> ("States Out"=w425:string)  [unwired: 14 in]
      }
      frame "UI: Initialize" {
        # "Initialize the User Interface, here.\n(this is called automatically, by the Macro: Init)"
        n199 = Unbundle By Name(w429) -> ("Core.Current VI Reference"=w428:refnum<vi>)
        n200 = property class="VI" props=["FP.Behavior"](reference=w428) -> ()  [unwired: 1 in, 3 out]
        n201 = local write "OK"(FALSE ("OK")) -> ()
        n202 = local write "Field/Temperature"(0 ("Field/Temperature")) -> ()
        n203 = local write "Tab Control"(T2."Intensity Graphs" ("Tab Control")) -> ()
        n204 = call <userlib>:"Fit VI window to Largest Dec__ogtk.vi"("error in (no error)"=w432, "border spacing (2 px)"=-2) -> ("error out"=w431:errorcluster)  [unwired: 4 in, 1 out]
        n205 = call <vilib>:"Add State(s) to Queue__jki_lib_state_machine.vi"("State(s) in (\"\")"=w436) -> ("States Out"=w435:string)  [unwired: 14 in]
      }
      frame "UI: Initialize Controls" {
        # "Do not put any code in this frame.\n(It is a separator no-op. You can make a copy of this frame to create a new UI frame)"
        n206 = Unbundle By Name(w438) -> ("INI"=w437:T13)
        n207 = Unbundle By Name(w437) -> ("Open DAT Path"=w453:path, "Export ITX Path"=w452:path, "Export ITX Name"=w451:string, "Intensity 1"=w450:T6, "X Offset 1"=w449:dbl, "derivative bin size 1"=w448:dbl, "e^2/h? 1"=w447:bool, "Log scale? 1"=w446:bool, "fake point 1"=w445:dbl, "Intensity 2"=w444:T6, "X Offset 2"=w443:dbl, "derivative bin size 2"=w442:dbl, "e^2/h? 2"=w441:bool, "Log scale? 2"=w440:bool, "fake point 2"=w439:dbl)
        n208 = local write "fake point 2"(w439) -> ()
        n209 = local write "Open DAT Path"(w453) -> ()
        n210 = local write "Export ITX Path"(w452) -> ()
        n211 = local write "Export ITX Name"(w451) -> ()
        n212 = local write "Intensity 1"(w450) -> ()
        n213 = local write "X Offset 1"(w449) -> ()
        n214 = local write "derivative bin size 1"(w448) -> ()
        n215 = local write "e^2/h? 1"(w447) -> ()
        n216 = local write "Log scale? 1"(w446) -> ()
        n217 = local write "fake point 1"(w445) -> ()
        n218 = local write "Intensity 2"(w444) -> ()
        n219 = local write "X Offset 2"(w443) -> ()
        n220 = local write "derivative bin size 2"(w442) -> ()
        n221 = local write "e^2/h? 2"(w441) -> ()
        n222 = local write "Log scale? 2"(w440) -> ()
        n223 = call <vilib>:"Add State(s) to Queue__jki_lib_state_machine.vi"("State(s) in (\"\")"=w456) -> ("States Out"=w455:string)  [unwired: 14 in]
      }
      frame "UI: Cursor Set" {
        # "Argument"
        # "Set and Unset Cursor Busy.\n(Usage: \"UI: Cursor Set >> Busy|Idle\")"
        n224 = case shown="\"Idle\", Default" w457 {
          tunnel: w459 -> [w464 w466]
          tunnel: [w463 w465] -> w458
          frame "Idle", Default {
            n225 = call <vilib>:"Unset Busy.vi"("error in (no error)"=w464) -> ("error out"=w463:errorcluster)  [unwired: 10 in]
          }
          frame "Busy" {
            n226 = call <vilib>:"Set Busy.vi"("error in (no error)"=w466) -> ("error out"=w465:errorcluster)  [unwired: 9 in, 1 out]
          }
        }
        n227 = call <vilib>:"Add State(s) to Queue__jki_lib_state_machine.vi"("State(s) in (\"\")"=w462) -> ("States Out"=w461:string)  [unwired: 14 in]
      }
      frame "UI: Front Panel State" {
        # "Argument"
        # "Set Front Panel Open or Closed\n(Usage: \"UI: Front Panel State >> Open|Close\")"
        n228 = Unbundle By Name(w469) -> ("Core.Current VI Reference"=w468:refnum<vi>)
        n229 = case shown="\"Minimize\", \"Minimized\"" w467 {
          tunnel: w471 -> [w479 w494 w505 w518 w531]
          tunnel: [w481 w495 w507 w520 w533] -> w470
          tunnel: w468 -> [w480 w492 w506 w519 w532]
          frame "Open", "Standard", Default {
            w474 = T11."Standard" ("State")
            n230 = property class="VI"(reference=w480, error in=w479) -> (reference out=w477:refnum<vi>, error out=w478:errorcluster, "FP.State"=w476:T11)
            n231 = Not Equal?(x=w476, y=w474) -> (x != y?=w475:bool)
            n232 = case shown="True" w475 {
              tunnel: [w485 w487] -> w481
              tunnel: w478 -> [w484 w487]
              tunnel: w477 -> [w483 _]
              tunnel: w474 -> [w482 _]
              frame True {
                n233 = invoke class="VI" method="FP.Open"(reference=w483, error in=w484, "Activate"=TRUE, "State"=w482) -> (error out=w485:errorcluster)  [unwired: 1 in, 4 out]
              }
              frame False {
              }
            }
          }
          frame "Close", "Closed" {
            n234 = property class="VI"(reference=w492, error in=w494) -> (reference out=w491:refnum<vi>, error out=w493:errorcluster, "FP.State"=w489:T11)
            n235 = Not Equal?(x=w489, y=T11."Closed" ("Front Panel Window:State")) -> (x != y?=w488:bool)
            n236 = case shown="True" w488 {
              tunnel: [w496 w499] -> w495
              tunnel: w493 -> [w496 w498]
              tunnel: w491 -> [_ w497]
              frame False {
              }
              frame True {
                n237 = invoke class="VI" method="FP.Close"(reference=w497, error in=w498) -> (error out=w499:errorcluster)  [unwired: 1 in, 2 out]
              }
            }
          }
          frame "Hidden", "Hide" {
            w500 = T11."Hidden" ("State")
            n238 = property class="VI"(reference=w506, error in=w505) -> (reference out=w503:refnum<vi>, error out=w504:errorcluster, "FP.State"=w502:T11)
            n239 = Not Equal?(x=w502, y=w500) -> (x != y?=w501:bool)
            n240 = case shown="True" w501 {
              tunnel: [w511 w512] -> w507
              tunnel: w504 -> [w510 w512]
              tunnel: w503 -> [w509 _]
              tunnel: w500 -> [w508 _]
              frame True {
                n241 = invoke class="VI" method="FP.Open"(reference=w509, error in=w510, "State"=w508) -> (error out=w511:errorcluster)  [unwired: 2 in, 4 out]
              }
              frame False {
              }
            }
          }
          frame "Minimize", "Minimized" {
            w513 = T11."Minimized" ("State")
            n242 = property class="VI"(reference=w519, error in=w518) -> (reference out=w516:refnum<vi>, error out=w517:errorcluster, "FP.State"=w515:T11)
            n243 = Not Equal?(x=w515, y=w513) -> (x != y?=w514:bool)
            n244 = case shown="True" w514 {
              tunnel: [w524 w525] -> w520
              tunnel: w517 -> [w523 w525]
              tunnel: w516 -> [w522 _]
              tunnel: w513 -> [w521 _]
              frame True {
                n245 = invoke class="VI" method="FP.Open"(reference=w522, error in=w523, "State"=w521) -> (error out=w524:errorcluster)  [unwired: 2 in, 4 out]
              }
              frame False {
              }
            }
          }
          frame "Maximize", "Maximized" {
            w526 = T11."Maximized" ("State")
            n246 = property class="VI"(reference=w532, error in=w531) -> (reference out=w529:refnum<vi>, error out=w530:errorcluster, "FP.State"=w528:T11)
            n247 = Not Equal?(x=w528, y=w526) -> (x != y?=w527:bool)
            n248 = case shown="True" w527 {
              tunnel: [w537 w538] -> w533
              tunnel: w530 -> [w536 w538]
              tunnel: w529 -> [w535 _]
              tunnel: w526 -> [w534 _]
              frame True {
                n249 = invoke class="VI" method="FP.Open"(reference=w535, error in=w536, "State"=w534) -> (error out=w537:errorcluster)  [unwired: 2 in, 4 out]
              }
              frame False {
              }
            }
          }
        }
        n250 = call <vilib>:"Add State(s) to Queue__jki_lib_state_machine.vi"("State(s) in (\"\")"=w473) -> ("States Out"=w472:string)  [unwired: 14 in]
      }
      frame "UI: Choose Tab" {
        # "Do not put any code in this frame.\n(It is a separator no-op. You can make a copy of this frame to create a new UI frame)"
        n251 = case shown="\"Intensity Graphs\", Default" w540 {
          tunnel: [T2."Intensity Graphs" ("Value (Signaling)")] -> w539
          frame "Intensity Graphs", Default {
          }
        }
        n252 = disable-structure shown="Disabled" {
          frame Disabled {
            n253 = property on="Tab Control" class="TabCtl (strict)"() -> ("Pages"=w545:refnum<vi>[])  [unwired: 2 in, 2 out]
            n254 = for {
              tunnel: w545 -> [w547] mode=indexing
              tunnel: [w546] -> _ mode=indexing
              n255 = property class="Page"(reference=w547) -> ("PageLabel"=w546:string)  [unwired: 1 in, 2 out]
            }
          }
          frame Enabled {
          }
        }
        n256 = property on="Tab Control" class="TabCtl (strict)"("Val(Sgnl)"=w539) -> ()  [unwired: 2 in, 2 out]
        n257 = call <vilib>:"Add State(s) to Queue__jki_lib_state_machine.vi"("State(s) in (\"\")"=w544) -> ("States Out"=w543:string)  [unwired: 14 in]
      }
      frame "---------- Macro ----------" {
        # "Do not put any code in this frame.\n(It is a separator no-op. You can make a copy of this frame to create a new Macro frame)"
        n258 = call <vilib>:"Add State(s) to Queue__jki_lib_state_machine.vi"("State(s) in (\"\")"=w552) -> ("States Out"=w551:string)  [unwired: 14 in]
      }
      frame "Macro: Initialize" {
        # "Initialization Macro\n(This is called once, when the VI starts)"
        n259 = call <vilib>:"Add State(s) to Queue__jki_lib_state_machine.vi"("State(s) in Front (\"\")"="Data: Initialize\nInitialize Core Data\nUI: Initialize\nUI: Front Panel State >> Open\n\nData: Read INI\nUI: Initialize Controls\n\nGraph: Initialize\nData Visualize: Initialize DVRs", "State(s) in (\"\")"=w557) -> ("States Out"=w556:string)  [unwired: 13 in]
      }
      frame "Macro: Exit" {
        # "Exit Macro\n(This is called once, when the VI exits)"
        n260 = Unbundle By Name(w565) -> ("Core.Close Panel on Exit?"=w564:bool)
        n261 = Select(t="UI: Front Panel State >> Close", s=w564, f="") -> (s? t:f=w561:string)
        n262 = call <vilib>:"Add State(s) to Queue__jki_lib_state_machine.vi"("State(s) in Front (\"\")"="Data: Write INI\nData Visualize: Cleanup DVRs", "State(s) in (\"\")"=w561, "State(s) at Back (\"\")"="Data: Cleanup\nExit") -> ("States Out"=w559:string)  [unwired: 12 in]
        n263 = call <vilib>:"Add State(s) to Queue__jki_lib_state_machine.vi"("State(s) in Front (\"\")"=w559, "State(s) in (\"\")"=w568) -> ("States Out"=w567:string)  [unwired: 13 in]
      }
      frame "Macro: Update Graphs" {
        # "Do not put any code in this frame.\n(It is a separator no-op. You can make a copy of this frame to create a new Macro frame)"
        n264 = call <vilib>:"Add State(s) to Queue__jki_lib_state_machine.vi"("State(s) in (\"\")"=w572) -> ("States Out"=w571:string)  [unwired: 14 in]
      }
      frame "Macro: Visualize" {
        # "Do not put any code in this frame.\n(It is a separator no-op. You can make a copy of this frame to create a new Macro frame)"
        n265 = call <vilib>:"Add State(s) to Queue__jki_lib_state_machine.vi"("State(s) in Front (\"\")"="Data Visualize: Read DAT File\nData Visualize: Cleanup DVRs\nData Visualize: Initialize DVRs\nData Visualize: Initialize Cursor Graph\nData Visualize: Calculate Derivative\n//Data Visualize: SG Filter\nData Visualize: Calculate Indices\nGraph: Initialize\nGraph: Set Y\nGraph: Set Labels\n//Data Visualize: Calculate Indices\n//Data Visualize: Choose Data 1\n//Data Visualize: Choose Data 2\n//Graph: Linecuts\nUI: Choose Tab >> Intensity Graphs\nUI: Cursor Set >> Idle" ("State(s) in Front (\"\")"), "State(s) in (\"\")"=w577) -> ("States Out"=w576:string)  [unwired: 13 in]
      }
      frame "Macro: Generate" {
        # "Do not put any code in this frame.\n(It is a separator no-op. You can make a copy of this frame to create a new Macro frame)"
        n266 = call <vilib>:"Add State(s) to Queue__jki_lib_state_machine.vi"("State(s) in Front (\"\")"="Data Generation: Update Class Wire\nData Generation: Read ITX Files\nData Generation: Write DAT File" ("State(s) in Front (\"\")"), "State(s) in (\"\")"=w582) -> ("States Out"=w581:string)  [unwired: 13 in]
      }
      frame "---------- Data Generation ----------" {
        # "Template Separator\n(You can make a copy of, or modify, this frame)"
        n267 = call <vilib>:"Add State(s) to Queue__jki_lib_state_machine.vi"("State(s) in (\"\")"=w586) -> ("States Out"=w585:string)  [unwired: 14 in]
      }
      frame "Data Generation: Update Class Wire" {
        # "Template Separator\n(You can make a copy of, or modify, this frame)"
        n268 = Unbundle By Name(w594) -> ("Retrieve and Visualize"=w596:refnum<class "Retrieve and Visualize.lvclass">)
        n269 = Bundle By Name(cluster=w596, "File or Folder Path"="Path", "T/B third axis"="T/B third axis", "IV setup"="IV setup", "index"="index", "Portion of data"="Portion of data", "Decimate point"="Decimate point", "Parameters from comments?"="Extract paramaters from comments?", "Scan names"="Scan names") -> (w595:refnum<class "Retrieve and Visualize.lvclass">)
        n270 = Bundle By Name(cluster=w594, "Retrieve and Visualize"=w595) -> (w593:T14)
        n271 = call <vilib>:"Add State(s) to Queue__jki_lib_state_machine.vi"("State(s) in (\"\")"=w601) -> ("States Out"=w600:string)  [unwired: 14 in]
      }
      frame "Data Generation: Read ITX Files" {
        # "Your code here.\n(You can make a copy of, or modify, this frame)"
        n272 = Unbundle By Name(w607) -> ("Retrieve and Visualize"=w608:refnum<class "Retrieve and Visualize.lvclass">)
        n273 = for {
          N: "# of fields/Temperatures" -> [w616]
          shift-right: [w623] -> w605
          shift-left: w608 -> [w620]
          tunnel: [w613] -> w603
          tunnel: w604 -> [w612]
          i -> [w615]
          n274 = Multiply(x=w615, y="Field Period") -> (x*y=w619:i32)
          n275 = Bundle By Name(cluster=w620, "# of B/T"=w616, "B/T offset"=w619, "Field Period"="Field Period") -> (w617:refnum<class "Retrieve and Visualize.lvclass">)
          n276 = call "Data retrieve engine_SE.vi"("error in (no error)"=w612, "File Type"="File Type", "Retrieve and Visualize"=w617) -> ("error out"=w622:errorcluster, "Retrieve and Visualize out"=w621:refnum<class "Retrieve and Visualize.lvclass">)  [unwired: 7 in]
          n277 = call "Create DAT Comments.vi"("error in"=w622, "Additional comments"="Additional comments", "Retrieve and Visualize"=w621) -> ("error out"=w613:errorcluster, "Retrieve and Visualize out"=w623:refnum<class "Retrieve and Visualize.lvclass">)  [unwired: 7 in]
        }
        n278 = Bundle By Name(cluster=w607, "Retrieve and Visualize"=w605) -> (w606:T14)
        n279 = call <vilib>:"Add State(s) to Queue__jki_lib_state_machine.vi"("State(s) in (\"\")"=w610) -> ("States Out"=w609:string)  [unwired: 14 in]
      }
      frame "Data Generation: Check Files" {
        # "Template Separator\n(You can make a copy of, or modify, this frame)"
        n280 = local read "Path"() -> (w629:path)
        n281 = local read "index"() -> (w628:T4)
        n282 = local read "File Type"() -> (w627:T5)
        n283 = call "LV to ITX Retrieve_SE mode.vi"("File or Folder Path"=w629, "offset"=0, "length"=1, "index"=w628, "stop"=FALSE, "File Type"=w627) -> ()  [unwired: 10 out]
        n284 = call <vilib>:"Add State(s) to Queue__jki_lib_state_machine.vi"("State(s) in (\"\")"=w633) -> ("States Out"=w632:string)  [unwired: 14 in]
      }
      frame "Data Generation: Write DAT File" {
        # "Your code here.\n(You can make a copy of, or modify, this frame)"
        n285 = Unbundle By Name(w637) -> ("Retrieve and Visualize"=w636:refnum<class "Retrieve and Visualize.lvclass">)
        n286 = call "Create DAT File.vi"("error in"=w639, "IV file name"="IV file name", "Processed data folder"="DAT folder", "Retrieve and Visualize"=w636) -> ("error out"=w638:errorcluster)  [unwired: 6 in, 1 out]
        n287 = call <vilib>:"Add State(s) to Queue__jki_lib_state_machine.vi"("State(s) in (\"\")"=w641) -> ("States Out"=w640:string)  [unwired: 14 in]
      }
      frame "---------- Data Visualize ----------" {
        # "Template Separator\n(You can make a copy of, or modify, this frame)"
        n288 = call <vilib>:"Add State(s) to Queue__jki_lib_state_machine.vi"("State(s) in (\"\")"=w645) -> ("States Out"=w644:string)  [unwired: 14 in]
      }
      frame "Data Visualize: Read DAT File" {
        # "Template Separator\n(You can make a copy of, or modify, this frame)"
        n289 = Empty String/Path?(string/path="Open DAT Path") -> (empty?=w651:bool)
        n290 = call-poly <userlib>:"File Exists__ogtk.vi"("file path"="Open DAT Path") -> ("exists"=w653:bool)  [unwired: 6 in, 1 out]
        n291 = Not(x=w653) -> (.not. x?=w652:bool)
        n292 = Or(x=w651, y=w652) -> ()  [unwired: 1 out]
        n293 = call <vilib>:"Get File Extension.vi"("error in (no error)"=w647, "file"="Open DAT Path") -> ("error out"=w646:errorcluster, "lowercase file extension"=w650:string, "dup file"=w648:path)  [unwired: 5 in, 2 out]
        n294 = case shown="\"dat\"" w650 {
          tunnel: [w663 w666] -> w654
          tunnel: w648 -> [w663 _]
          tunnel: w646 -> [w662 w668]
          tunnel: [w662 w667] -> w655
          frame "dat" {
          }
          frame Default {
            w664 = "DAT" ("pattern label")
            n295 = call "File Dialog"("button label"=w664, "error in"=w668, "pattern (all files)"="*.dat", "pattern label"=w664) -> ("selected path"=w666:path, "error out"=w667:errorcluster)  [unwired: 8 in, 2 out]
          }
        }
        n296 = call "Read DAT File.vi"("error in"=w655, "file path (use dialog)"=w654) -> ("error out"=w659:errorcluster, "Retrieve and Visualize out"=w658:refnum<class "Retrieve and Visualize.lvclass">)  [unwired: 8 in]
        n297 = local write "Open DAT Path"(w654) -> ()
        n298 = Bundle By Name(cluster=w657, "Retrieve and Visualize"=w658) -> (w656:T14)
        n299 = call <vilib>:"Add State(s) to Queue__jki_lib_state_machine.vi"("State(s) in (\"\")"=w661) -> ("States Out"=w660:string)  [unwired: 14 in]
      }
      frame "Data Visualize: Initialize DVRs" {
        w670 = cluster{dbl[], dbl[]}[][][] [] ("DAT File.IV-2T")
        # "Template Separator\n(You can make a copy of, or modify, this frame)"
        n300 = Unbundle By Name(w690) -> ("Retrieve and Visualize"=w691:refnum<class "Retrieve and Visualize.lvclass">)
        n301 = Unbundle By Name(w691) -> ("IV"=w692:cluster{dbl[], dbl[]}[][][], "IV-2T"=w676:cluster{dbl[], dbl[]}[][][], "Vfast"=w686:dbl[][], "Vslow"=w685:dbl[], "Vslowest"=w684:dbl[], "Comments"=→"Comments":string, "Scan names"=w669:string[])
        n302 = New Data Value Reference(data value=w692, error in=w683) -> (data value reference=w688:refnum<data-value>, error out=w681:errorcluster)
        n303 = New Data Value Reference(data value=w676, error in=w681) -> (data value reference=w687:refnum<data-value>, error out=w680:errorcluster)
        n304 = New Data Value Reference(data value=w670, error in=w680) -> (data value reference=w672:refnum<data-value>, error out=w679:errorcluster)
        n305 = New Data Value Reference(data value=w670, error in=w679) -> (data value reference=w673:refnum<data-value>, error out=w678:errorcluster)
        n306 = New Data Value Reference(data value=w670, error in=w678) -> (data value reference=w674:refnum<data-value>, error out=w677:errorcluster)
        n307 = New Data Value Reference(data value=w670, error in=w677) -> (data value reference=w675:refnum<data-value>, error out=w682:errorcluster)
        n308 = Bundle By Name(cluster=w690, "DVR.IV-4T"=w688, "DVR.IV-2T"=w687, "DVR.G-4T"=w672, "DVR.R-4T"=w673, "DVR.G-2T"=w674, "DVR.R-2T"=w675, "Vfast"=w686, "Vslow"=w685, "Vslowest"=w684, "Scan Names"=w669) -> (w689:T14)
        n309 = call <vilib>:"Add State(s) to Queue__jki_lib_state_machine.vi"("State(s) in (\"\")"=w694) -> ("States Out"=w693:string)  [unwired: 14 in]
      }
      frame "Data Visualize: Cleanup DVRs" {
        # "Template Separator\n(You can make a copy of, or modify, this frame)"
        n310 = Unbundle By Name(w699) -> ("DVR"=w698:T16)
        n311 = Unbundle By Name(w698) -> ("IV-4T"=w696:refnum<data-value>, "G-2T"=w710:refnum<data-value>, "R-2T"=w709:refnum<data-value>, "G-4T"=w708:refnum<data-value>, "R-4T"=w707:refnum<data-value>, "IV-2T"=w706:refnum<data-value>)
        n312 = Delete Data Value Reference(data value reference=w706) -> (error out=w705:errorcluster)  [unwired: 1 in, 1 out]
        n313 = Delete Data Value Reference(data value reference=w707) -> (error out=w700:errorcluster)  [unwired: 1 in, 1 out]
        n314 = Delete Data Value Reference(data value reference=w708) -> (error out=w701:errorcluster)  [unwired: 1 in, 1 out]
        n315 = Delete Data Value Reference(data value reference=w709) -> (error out=w702:errorcluster)  [unwired: 1 in, 1 out]
        n316 = Delete Data Value Reference(data value reference=w710) -> (error out=w703:errorcluster)  [unwired: 1 in, 1 out]
        n317 = Delete Data Value Reference(data value reference=w696) -> (error out=w704:errorcluster)  [unwired: 1 in, 1 out]
        n318 = Merge Errors(w704, w703, w702, w701, w700, w705) -> (w695:errorcluster)
        n319 = disable-structure shown="Enabled" {
          disable-tunnel: w695 -> [w713 _]
          frame Disabled {
            n320 = flat-sequence {
              tunnel: w713 -> [_]
              frame #0 {
                n321 = Request Deallocation(TRUE ("flag")) -> ()
              }
            }
          }
          frame Enabled {
          }
        }
        n322 = call <vilib>:"Clear Errors.vi"("error in (no error)"=w695) -> ("error out"=w697:errorcluster)  [unwired: 5 in, 1 out]
        n323 = call <vilib>:"Add State(s) to Queue__jki_lib_state_machine.vi"("State(s) in (\"\")"=w712) -> ("States Out"=w711:string)  [unwired: 14 in]
      }
      frame "Data Visualize: Initialize Cursor Graph" {
        w719 = dbl[] []
        # "Initialize Cursor Graph"
        # "replace with array resize?"
        # "Do not put any code in this frame.\n(It is a separator no-op. You can make a copy of this frame to create a new UI frame)"
        n324 = Unbundle By Name(w715) -> ("Vfast"=w721:dbl[][], "Vslow"=w720:dbl[], "Scan Names"=w725:string[])
        n325 = Transpose 2D Array(2D array=w721) -> (transposed array=w716:dbl[][])
        n326 = for {
          tunnel: w716 -> [w734] mode=indexing
          tunnel: w720 -> [w731]
          shift-right: [w732] -> w722
          shift-left: w719 -> [w733]
          shift-right: [w730] -> w723
          shift-left: w719 -> [w729]
          n327 = Build Array (concatenate)(w733, w734) -> (w732:dbl[])
          n328 = Build Array (concatenate)(w729, w731) -> (w730:dbl[])
        }
        n329 = Index Array(array=w725) -> (element #1=w717:string, element #2=w724:string)  [unwired: 2 in]
        n330 = property on="Cursor Graph" class="XYGraph (strict)"("XScale.NameLbl.Text"=w717, "YScale.NameLbl.Text"=w724) -> ()  [unwired: 2 in, 2 out]
        n331 = Bundle(w722, w723) -> (→"Cursor Graph":cluster{dbl[], dbl[]})  [unwired: 1 in]
        n332 = call <vilib>:"Add State(s) to Queue__jki_lib_state_machine.vi"("State(s) in (\"\")"=w728) -> ("States Out"=w727:string)  [unwired: 14 in]
      }
      frame "Data Visualize: Calculate Derivative" {
        w741 = enum16{"dy/dx vs x", "dx/dy vs y"}."dy/dx vs x" ("Type")
        w742 = enum16{"dy/dx vs x", "dx/dy vs y"}."dx/dy vs y" ("Type")
        # "Template Separator\n(You can make a copy of, or modify, this frame)"
        n333 = Unbundle By Name(w754) -> ("DVR.IV-4T"=w736:refnum<data-value>, "DVR.G-4T"=w740:refnum<data-value>, "DVR.R-4T"=w739:refnum<data-value>, "DVR.IV-2T"=w735:refnum<data-value>, "DVR.G-2T"=w738:refnum<data-value>, "DVR.R-2T"=w737:refnum<data-value>)
        n334 = call "Derivative (DVR).vi"("Type"=w742, "Fit Points"="Fit Points", "Data Value Reference in"=w736, "error in (no error)"=w745, "dX in"=w740) -> ("error out"=w748:errorcluster, "dX out"=w749:refnum<data-value>)  [unwired: 5 in]
        n335 = call "Derivative (DVR).vi"("Type"=w741, "Fit Points"="Fit Points", "Data Value Reference in"=w736, "error in (no error)"=w748, "dX in"=w739) -> ("error out"=w747:errorcluster, "dX out"=w750:refnum<data-value>)  [unwired: 5 in]
        n336 = call "Derivative (DVR).vi"("Type"=w742, "Fit Points"="Fit Points", "Data Value Reference in"=w735, "error in (no error)"=w747, "dX in"=w738) -> ("error out"=w746:errorcluster, "dX out"=w751:refnum<data-value>)  [unwired: 5 in]
        n337 = call "Derivative (DVR).vi"("Type"=w741, "Fit Points"="Fit Points", "Data Value Reference in"=w735, "error in (no error)"=w746, "dX in"=w737) -> ("error out"=w744:errorcluster, "dX out"=w752:refnum<data-value>)  [unwired: 5 in]
        n338 = Bundle By Name(cluster=w754, "DVR.G-4T"=w749, "DVR.R-4T"=w750, "DVR.G-2T"=w751, "DVR.R-2T"=w752) -> (w753:T14)
        n339 = call <vilib>:"Add State(s) to Queue__jki_lib_state_machine.vi"("State(s) in (\"\")"=w756) -> ("States Out"=w755:string)  [unwired: 14 in]
      }
      frame "Data Visualize: SG Filter" {
        # "Template Separator\n(You can make a copy of, or modify, this frame)"
        n340 = Unbundle By Name(w771) -> ("DVR.G-2T"=w773:refnum<data-value>, "DVR.R-2T"=w769:refnum<data-value>, "DVR.G-4T"=w768:refnum<data-value>, "DVR.R-4T"=w767:refnum<data-value>)
        n341 = call "SG Filter (DVR).vi"("error in"=w763, "side points"="side points 2T", "Data Value Reference in"=w773) -> ("error out"=w762:errorcluster, "Data Value Reference out"=w772:refnum<data-value>)  [unwired: 7 in]
        n342 = call "SG Filter (DVR).vi"("error in"=w762, "side points"="side points 2T", "Data Value Reference in"=w769) -> ("error out"=w761:errorcluster, "Data Value Reference out"=w766:refnum<data-value>)  [unwired: 7 in]
        n343 = call "SG Filter (DVR).vi"("error in"=w761, "side points"="side points 4T", "Data Value Reference in"=w768) -> ("error out"=w760:errorcluster, "Data Value Reference out"=w765:refnum<data-value>)  [unwired: 7 in]
        n344 = call "SG Filter (DVR).vi"("error in"=w760, "side points"="side points 4T", "Data Value Reference in"=w767) -> ("error out"=w759:errorcluster, "Data Value Reference out"=w764:refnum<data-value>)  [unwired: 7 in]
        n345 = Bundle By Name(cluster=w771, "DVR.G-2T"=w772, "DVR.R-2T"=w766, "DVR.G-4T"=w765, "DVR.R-4T"=w764) -> (w770:T14)
        n346 = call <vilib>:"Add State(s) to Queue__jki_lib_state_machine.vi"("State(s) in (\"\")"=w775) -> ("States Out"=w774:string)  [unwired: 14 in]
      }
      frame "Data Visualize: Calculate Indices" {
        # "used?"
        # "used?"
        # "used?"
        # "used?"
        # "Calculate Indices"
        # "Template Separator\n(You can make a copy of, or modify, this frame)"
        n347 = Unbundle By Name(w786) -> ("Vfast"=w789:dbl[][], "Vslow"=w788:dbl[], "Vslowest"=w787:dbl[])
        n348 = property on="Cursor Graph" class="XYGraph (strict)"(error in=w777) -> (error out=w776:errorcluster, "Cursor.Cursor X"=w795:dbl, "Cursor.Cursor Y"=w794:dbl)  [unwired: 1 in, 1 out]
        "Slow" <- w794
        "Fast" <- w795
        n349 = local read "Field/Temperature"() -> (w792:i32)
        n350 = Index Array(array=w787, index=w792) -> (element=→"slowest":dbl)
        n351 = call "Calculate Indices.vi"("Cursor.Cursor Y"=w794, "Cursor.Cursor X"=w795, "Vslow"=w788, "Vfast"=w789) -> ("Column"=w778:i32, "Row"=w779:i32, "Column Array"=w780:i32[], "Row Array"=w781:i32[])  [unwired: 4 in]
        n352 = Array Size(array=w787) -> (size(s)=w790:i32)
        n353 = Decrement(x=w790) -> (x-1=w791:i32)
        n354 = Index Array(array=w789, index (row)=w779) -> (element=w783:dbl[])  [unwired: 1 in]
        n355 = property on="Field/Temperature" class="Slide (strict)"("Scale.Maximum"=w791) -> ()  [unwired: 2 in, 2 out]
        n356 = Reverse 1D Array(array=w788) -> (reversed array=w784:dbl[])
        n357 = Bundle By Name(cluster=w786, "Vfast Slice"=w783, "Vslow Slice"=w784, "Page"="Field/Temperature", "Row Array"=w781, "Column Array"=w780, "Row"=w779, "Column"=w778) -> (w785:T14)
        n358 = call <vilib>:"Add State(s) to Queue__jki_lib_state_machine.vi"("State(s) in (\"\")"=w797) -> ("States Out"=w796:string)  [unwired: 14 in]
      }
      frame "Data Visualize: Vary Vfast" {
        # "Template Separator\n(You can make a copy of, or modify, this frame)"
        n359 = Unbundle By Name(w800) -> ("DVR.IV-4T"=w801:refnum<data-value>, "DVR.G-2T"=w806:refnum<data-value>, "DVR.R-2T"=w802:refnum<data-value>, "DVR.G-4T"=w803:refnum<data-value>, "DVR.R-4T"=w804:refnum<data-value>, "DVR.IV-2T"=w805:refnum<data-value>, "Page"=w798:i32, "Row"=w799:i32)
        n360 = in-place {
          in-place-border: w798 -> [w818]
          in-place-border: w799 -> [w816]
          n361 = in-place-dvr #3(w801) -> (w815:cluster{dbl[], dbl[]}[][][])  [unwired: 1 out]
          n362 = in-place-dvr #4(w806) -> (w814:cluster{dbl[], dbl[]}[][][])  [unwired: 1 out]
          n363 = in-place-dvr #5(w802) -> (w813:cluster{dbl[], dbl[]}[][][])  [unwired: 1 out]
          n364 = in-place-dvr #6(w803) -> (w812:cluster{dbl[], dbl[]}[][][])  [unwired: 1 out]
          n365 = in-place-dvr #7(w804) -> (w811:cluster{dbl[], dbl[]}[][][])  [unwired: 1 out]
          n366 = in-place-dvr #8(w805) -> (w810:cluster{dbl[], dbl[]}[][][])  [unwired: 1 out]
          n367 = Index Array(array=w815, index (dim 0)=w818) -> (element=w827:cluster{dbl[], dbl[]}[][])  [unwired: 2 in]
          n368 = Index Array(array=w814, index (dim 0)=w818) -> (element=w821:cluster{dbl[], dbl[]}[][])  [unwired: 2 in]
          n369 = Index Array(array=w813, index (dim 0)=w818, index (dim 1)=w816) -> (element=→"dV/dI 2T":cluster{dbl[], dbl[]}[])  [unwired: 1 in]
          n370 = Index Array(array=w812, index (dim 0)=w818) -> (element=w825:cluster{dbl[], dbl[]}[][])  [unwired: 2 in]
          n371 = Index Array(array=w811, index (dim 0)=w818, index (dim 1)=w816) -> (element=→"dV/dI":cluster{dbl[], dbl[]}[])  [unwired: 1 in]
          n372 = Index Array(array=w810, index (dim 0)=w818) -> (element=w823:cluster{dbl[], dbl[]}[][])  [unwired: 2 in]
          n373 = Index Array(array=w827, index (row)=w816) -> (element=→"IV":cluster{dbl[], dbl[]}[])  [unwired: 1 in]
          n374 = Index Array(array=w821, index (row)=w816) -> (element=→"dI/dV 2T":cluster{dbl[], dbl[]}[])  [unwired: 1 in]
          n375 = Index Array(array=w825, index (row)=w816) -> (element=→"dI/dV":cluster{dbl[], dbl[]}[])  [unwired: 1 in]
          n376 = Index Array(array=w823, index (row)=w816) -> (element=→"IV 2T":cluster{dbl[], dbl[]}[])  [unwired: 1 in]
          n377 = in-place-dvr #3(w815) -> ()  [unwired: 2 out]
          n378 = in-place-dvr #4(w814) -> ()  [unwired: 2 out]
          n379 = in-place-dvr #5(w813) -> ()  [unwired: 2 out]
          n380 = in-place-dvr #6(w812) -> ()  [unwired: 2 out]
          n381 = in-place-dvr #7(w811) -> ()  [unwired: 2 out]
          n382 = in-place-dvr #8(w810) -> ()  [unwired: 2 out]
        }
        n383 = call <vilib>:"Add State(s) to Queue__jki_lib_state_machine.vi"("State(s) in (\"\")"=w809) -> ("States Out"=w808:string)  [unwired: 14 in]
      }
      frame "Data Visualize: Vary Vslow" {
        # "col[]"
        # "row[]"
        # "page"
        # "Template Separator\n(You can make a copy of, or modify, this frame)"
        n384 = Unbundle By Name(w832) -> ("DVR"=w831:T16, "Page"=w828:i32, "Row Array"=w830:i32[], "Column Array"=w829:i32[])
        n385 = Unbundle By Name(w831) -> ("IV-4T"=w836:refnum<data-value>, "G-2T"=w835:refnum<data-value>, "G-4T"=w833:refnum<data-value>, "IV-2T"=w834:refnum<data-value>)
        n386 = in-place {
          in-place-border: w828 -> [w850]
          in-place-border: w830 -> [w845]
          in-place-border: w829 -> [w844]
          n387 = in-place-dvr #9(w836) -> (w843:cluster{dbl[], dbl[]}[][][])  [unwired: 1 out]
          n388 = in-place-dvr #10(w835) -> (w842:cluster{dbl[], dbl[]}[][][])  [unwired: 1 out]
          n389 = in-place-dvr #11(w833) -> (w841:cluster{dbl[], dbl[]}[][][])  [unwired: 1 out]
          n390 = in-place-dvr #12(w834) -> (w840:cluster{dbl[], dbl[]}[][][])  [unwired: 1 out]
          n391 = for {
            tunnel: w842 -> [w861]
            tunnel: w850 -> [w854]
            tunnel: w844 -> [w852] mode=indexing
            tunnel: [w860] -> w849 mode=indexing
            tunnel: w845 -> [w853] mode=indexing
            tunnel: w841 -> [w859]
            tunnel: [w858] -> w848 mode=indexing
            tunnel: w840 -> [w857]
            tunnel: [w856] -> w847 mode=indexing
            tunnel: w843 -> [w855]
            tunnel: [w851] -> w846 mode=indexing
            n392 = Index Array(array=w855, index (dim 0)=w854, index (dim 1)=w853, index (dim 2)=w852) -> (element=w851:cluster{dbl[], dbl[]})
            n393 = Index Array(array=w861, index (dim 0)=w854, index (dim 1)=w853, index (dim 2)=w852) -> (element=w860:cluster{dbl[], dbl[]})
            n394 = Index Array(array=w859, index (dim 0)=w854, index (dim 1)=w853, index (dim 2)=w852) -> (element=w858:cluster{dbl[], dbl[]})
            n395 = Index Array(array=w857, index (dim 0)=w854, index (dim 1)=w853, index (dim 2)=w852) -> (element=w856:cluster{dbl[], dbl[]})
          }
          "IV slow 4T" <- w846
          "dI/dV slow 4T" <- w848
          "dI/dV slow 2T" <- w849
          "IV slow 2T" <- w847
          n396 = in-place-dvr #9(w843) -> ()  [unwired: 2 out]
          n397 = in-place-dvr #10(w842) -> ()  [unwired: 2 out]
          n398 = in-place-dvr #11(w841) -> ()  [unwired: 2 out]
          n399 = in-place-dvr #12(w840) -> ()  [unwired: 2 out]
        }
        n400 = call <vilib>:"Add State(s) to Queue__jki_lib_state_machine.vi"("State(s) in (\"\")"=w839) -> ("States Out"=w838:string)  [unwired: 14 in]
      }
      frame "Data Visualize: Vary Fields" {
        # "column"
        # "row"
        # "Template Separator\n(You can make a copy of, or modify, this frame)"
        n401 = Unbundle By Name(w865) -> ("DVR"=w864:T16, "Row"=w863:i32, "Column"=w862:i32)
        n402 = Unbundle By Name(w864) -> ("IV-4T"=w866:refnum<data-value>, "G-2T"=w868:refnum<data-value>, "G-4T"=w867:refnum<data-value>, "IV-2T"=w869:refnum<data-value>)
        n403 = in-place {
          in-place-border: w863 -> [w873]
          in-place-border: w862 -> [w882]
          n404 = in-place-dvr #13(w866) -> (w877:cluster{dbl[], dbl[]}[][][])  [unwired: 1 out]
          n405 = in-place-dvr #14(w868) -> (w876:cluster{dbl[], dbl[]}[][][])  [unwired: 1 out]
          n406 = in-place-dvr #15(w867) -> (w875:cluster{dbl[], dbl[]}[][][])  [unwired: 1 out]
          n407 = in-place-dvr #16(w869) -> (w874:cluster{dbl[], dbl[]}[][][])  [unwired: 1 out]
          n408 = Index Array(array=w877, index (dim 1)=w873, index (dim 2)=w882) -> (element=→"IV vary 3rd 4T":cluster{dbl[], dbl[]}[])  [unwired: 1 in]
          n409 = Index Array(array=w876, index (dim 1)=w873, index (dim 2)=w882) -> (element=→"dI/dV vary 3rd 2T":cluster{dbl[], dbl[]}[])  [unwired: 1 in]
          n410 = Index Array(array=w875, index (dim 1)=w873, index (dim 2)=w882) -> (element=→"dI/dV vary 3rd 4T":cluster{dbl[], dbl[]}[])  [unwired: 1 in]
          n411 = Index Array(array=w874, index (dim 1)=w873, index (dim 2)=w882) -> (element=→"IV vary 3rd 2T":cluster{dbl[], dbl[]}[])  [unwired: 1 in]
          n412 = in-place-dvr #13(w877) -> ()  [unwired: 2 out]
          n413 = in-place-dvr #14(w876) -> ()  [unwired: 2 out]
          n414 = in-place-dvr #15(w875) -> ()  [unwired: 2 out]
          n415 = in-place-dvr #16(w874) -> ()  [unwired: 2 out]
        }
        n416 = call <vilib>:"Add State(s) to Queue__jki_lib_state_machine.vi"("State(s) in (\"\")"=w872) -> ("States Out"=w871:string)  [unwired: 14 in]
      }
      frame "Data Visualize: Choose Data 1" {
        # "Template Separator\n(You can make a copy of, or modify, this frame)"
        n417 = local read "Intensity 1"() -> (w894:T6)
        n418 = Unbundle By Name(w908) -> ("Vfast Slice"=w886:dbl[], "Graph.Intensity 1"=w903:refnum<class "graph_utilities.lvclass">, "DVR"=w907:T16, "Page"=w906:i32, "Row"=w904:i32)
        n419 = case shown="\"R-4T\"" w894 {
          tunnel: w907 -> [w920 w922 w924 w926 w928 w930 w932]
          tunnel: [w919 w921 w923 w925 w927 w929 w931] -> w905
          frame "IV-4T", Default {
            n420 = Unbundle By Name(w920) -> ("IV-4T"=w919:refnum<data-value>)
          }
          frame "IV-2T" {
            n421 = Unbundle By Name(w922) -> ("IV-2T"=w921:refnum<data-value>)
          }
          frame "R-4T" {
            n422 = Unbundle By Name(w924) -> ("R-4T"=w923:refnum<data-value>)
          }
          frame "G-4T" {
            n423 = Unbundle By Name(w926) -> ("G-4T"=w925:refnum<data-value>)
          }
          frame "R-2T" {
            n424 = Unbundle By Name(w928) -> ("R-2T"=w927:refnum<data-value>)
          }
          frame "G-2T" {
            n425 = Unbundle By Name(w930) -> ("G-2T"=w929:refnum<data-value>)
          }
          frame "dGdVsg-4T" {
            n426 = Unbundle By Name(w932) -> ("G-4T"=w931:refnum<data-value>)
          }
        }
        n427 = call "Slice Row (DVR).vi"("Fake Point (0)"="fake point 1", "error in (no error)"=w887, "Row"=w904, "Page"=w906, "Data Value Reference in"=w905) -> ("X-array"=w884:dbl[], "2D Array"=w900:dbl[][])  [unwired: 4 in, 1 out]
        n428 = call "G to e2h (2D).vi"("e^2/h?"="e^2/h? 1", "Array in"=w900) -> ("error out"=w895:errorcluster, "Array out"=w901:dbl[][])  [unwired: 8 in]
        n429 = Subtract(x=w884, y="X Offset 1") -> (x-y=w885:dbl[])
        n430 = call "Log (2D).vi"("error in (no error)"=w895, "Log scale?"="Log scale? 1", "Array in"=w901) -> ("error out"=w896:errorcluster, "Array out"=w899:dbl[][])  [unwired: 7 in]
        n431 = case shown="\"dGdVsg-4T\"" w894 {
          tunnel: w899 -> [w912 w918]
          tunnel: [w912 w917] -> w898
          tunnel: "derivative bin size 1" -> [_ w916]
          tunnel: w896 -> [w911 w915]
          tunnel: [w911 w914] -> w891
          tunnel: w886 -> [_ w913]
          frame Default {
          }
          frame "dGdVsg-4T" {
            n432 = call "Derivative (2D).vi"("error in (no error)"=w915, "derivative bin size"=w916, "Axis Array"=w913, "Conductance"=w918) -> ("error out"=w914:errorcluster, "Transconductance"=w917:dbl[][])  [unwired: 6 in]
          }
        }
        n433 = call <userlib>:"Set Intensity Graph Value.vi"("error in (no error)"=w891, "Value"=w898, "graph_utilities in"=w903) -> ("error out"=w890:errorcluster, "graph_utilities out"=w902:refnum<class "graph_utilities.lvclass">)  [unwired: 7 in]
        n434 = call <userlib>:"Set Intensity Graph X Scale Array.vi"("error in (no error)"=w890, "X Scale"=w885, "graph_utilities in"=w902) -> ("error out"=w889:errorcluster)  [unwired: 7 in, 1 out]
        n435 = call <vilib>:"Add State(s) to Queue__jki_lib_state_machine.vi"("State(s) in (\"\")"=w910) -> ("States Out"=w909:string)  [unwired: 14 in]
      }
      frame "Data Visualize: Choose Data 2" {
        # "Template Separator\n(You can make a copy of, or modify, this frame)"
        n436 = Unbundle By Name(w958) -> ("Vfast Slice"=w936:dbl[], "Graph.Intensity 2"=w953:refnum<class "graph_utilities.lvclass">, "DVR"=w957:T16, "Page"=w956:i32, "Row"=w954:i32)
        n437 = local read "Intensity 2"() -> (w937:T6)
        n438 = case shown="\"dGdVsg-4T\"" w937 {
          tunnel: w957 -> [w970 w972 w974 w976 w978 w980 w982]
          tunnel: [w969 w971 w973 w975 w977 w979 w981] -> w955
          frame "IV-4T", Default {
            n439 = Unbundle By Name(w970) -> ("IV-4T"=w969:refnum<data-value>)
          }
          frame "IV-2T" {
            n440 = Unbundle By Name(w972) -> ("IV-2T"=w971:refnum<data-value>)
          }
          frame "R-4T" {
            n441 = Unbundle By Name(w974) -> ("R-4T"=w973:refnum<data-value>)
          }
          frame "G-4T" {
            n442 = Unbundle By Name(w976) -> ("G-4T"=w975:refnum<data-value>)
          }
          frame "R-2T" {
            n443 = Unbundle By Name(w978) -> ("R-2T"=w977:refnum<data-value>)
          }
          frame "G-2T" {
            n444 = Unbundle By Name(w980) -> ("G-2T"=w979:refnum<data-value>)
          }
          frame "dGdVsg-4T" {
            n445 = Unbundle By Name(w982) -> ("G-4T"=w981:refnum<data-value>)
          }
        }
        n446 = call "Slice Row (DVR).vi"("Fake Point (0)"="fake point 2", "error in (no error)"=w938, "Row"=w954, "Page"=w956, "Data Value Reference in"=w955) -> ("X-array"=w935:dbl[], "2D Array"=w950:dbl[][])  [unwired: 4 in, 1 out]
        n447 = call "G to e2h (2D).vi"("e^2/h?"="e^2/h? 2", "Array in"=w950) -> ("error out"=w945:errorcluster, "Array out"=w951:dbl[][])  [unwired: 8 in]
        n448 = Subtract(x=w935, y="X Offset 2") -> (x-y=w934:dbl[])
        n449 = call "Log (2D).vi"("error in (no error)"=w945, "Log scale?"="Log scale? 2", "Array in"=w951) -> ("error out"=w946:errorcluster, "Array out"=w949:dbl[][])  [unwired: 7 in]
        n450 = case shown="\"dGdVsg-4T\"" w937 {
          tunnel: w949 -> [w962 w968]
          tunnel: [w962 w967] -> w948
          tunnel: "derivative bin size 2" -> [_ w966]
          tunnel: w946 -> [w961 w965]
          tunnel: [w961 w964] -> w942
          tunnel: w936 -> [_ w963]
          frame Default {
          }
          frame "dGdVsg-4T" {
            n451 = call "Derivative (2D).vi"("error in (no error)"=w965, "derivative bin size"=w966, "Axis Array"=w963, "Conductance"=w968) -> ("error out"=w964:errorcluster, "Transconductance"=w967:dbl[][])  [unwired: 6 in]
          }
        }
        n452 = call <userlib>:"Set Intensity Graph Value.vi"("error in (no error)"=w942, "Value"=w948, "graph_utilities in"=w953) -> ("error out"=w941:errorcluster, "graph_utilities out"=w952:refnum<class "graph_utilities.lvclass">)  [unwired: 7 in]
        n453 = call <userlib>:"Set Intensity Graph X Scale Array.vi"("error in (no error)"=w941, "X Scale"=w934, "graph_utilities in"=w952) -> ("error out"=w940:errorcluster)  [unwired: 7 in, 1 out]
        n454 = call <vilib>:"Add State(s) to Queue__jki_lib_state_machine.vi"("State(s) in (\"\")"=w960) -> ("States Out"=w959:string)  [unwired: 14 in]
      }
      frame "---------- Data Export ----------" {
        # "Template Separator\n(You can make a copy of, or modify, this frame)"
        n455 = call <vilib>:"Add State(s) to Queue__jki_lib_state_machine.vi"("State(s) in (\"\")"=w986) -> ("States Out"=w985:string)  [unwired: 14 in]
      }
      frame "Data Export: Export" {
        # "Template Separator\n(You can make a copy of, or modify, this frame)"
        n456 = Unbundle By Name(w993) -> ("Graph"=w992:T15)
        n457 = case shown="\"Intensity 1\", Default" "Export What?" {
          selector: "Export What?" -> [w996 w1010 w1027 w1043 w1062 w1081]
          tunnel: w992 -> [w1008 w1025 w1042 w1055 w1072 w1089]
          tunnel: w989 -> [w1005 w1015 w1034 w1051 w1058 w1074]
          tunnel: [w1003 w1022 w1039 w1050 w1069 w1086] -> w991
          tunnel: "Export ITX Path" -> [w1000 w1013 w1030 w1045 w1068 w1080]
          tunnel: "Export ITX Name" -> [w999 w1014 w1029 w1046 w1064 w1083]
          frame "Intensity 1", Default {
            n458 = local read "Intensity 1"() -> (w997:T6)
            n459 = Format Into String(format string="%s-%s-%s-", w999, w997, w996) -> (resulting string=w1002:string)  [unwired: 2 in, 1 out]
            n460 = Unbundle By Name(w1008) -> ("Intensity 1"=w1007:refnum<class "graph_utilities.lvclass">)
            n461 = Build Path(base path=w1000, name or relative path=w1002) -> (appended path=w998:path)
            n462 = call <userlib>:"Read Intensity Graph ref.vi"("error in (no error)"=w1005, "graph_utilities in"=w1007) -> ("error out"=w1004:errorcluster, "Intensity Graph"=w1006:refnum<vi>)  [unwired: 6 in, 2 out]
            n463 = call <userlib>:"Intensity Graph to Igor Graph.vi"("error in (no error)"=w1004, "Intensity Graph Reference"=w1006, "Path"=w998) -> ("error out"=w1003:errorcluster)  [unwired: 7 in, 1 out]
          }
          frame "H Cut 1" {
            n464 = local read "Intensity 1"() -> (w1009:T6)
            n465 = Unbundle By Name(w1025) -> ("H 1"=w1018:refnum<class "graph_utilities.lvclass">)
            n466 = call <userlib>:"Get Intensity Graph Cursor (Control).vi"("error in (no error)"=w1015, "graph_utilities in"=w1018) -> ("error out"=w1016:errorcluster, "Cursor.Cursor Position"=w1019:T19, "graph_utilities out"=w1017:refnum<class "graph_utilities.lvclass">)  [unwired: 7 in]
            n467 = Unbundle By Name(w1019) -> ("Y"=w1011:dbl)
            n468 = Format Into String(format string="%s-%s-%s-%f-", w1014, w1009, w1010, w1011) -> (resulting string=w1021:string)  [unwired: 2 in, 1 out]
            n469 = call <userlib>:"Read XY Graph ref.vi"("error in (no error)"=w1016, "graph_utilities in"=w1017) -> ("error out"=w1024:errorcluster, "XY Graph"=w1023:refnum<vi>)  [unwired: 6 in, 2 out]
            n470 = Build Path(base path=w1013, name or relative path=w1021) -> (appended path=w1012:path)
            n471 = call <userlib>:"XY Graph to Igor Graph.vi"("error in (no error)"=w1024, "XY Graph Reference"=w1023, "Path"=w1012) -> ("error out"=w1022:errorcluster)  [unwired: 7 in, 1 out]
          }
          frame "V Cut 1" {
            n472 = local read "Intensity 1"() -> (w1026:T6)
            n473 = Unbundle By Name(w1042) -> ("V 1"=w1035:refnum<class "graph_utilities.lvclass">)
            n474 = call <userlib>:"Get Intensity Graph Cursor (Control).vi"("error in (no error)"=w1034, "graph_utilities in"=w1035) -> ("error out"=w1032:errorcluster, "Cursor.Cursor Position"=w1036:T19, "graph_utilities out"=w1033:refnum<class "graph_utilities.lvclass">)  [unwired: 7 in]
            n475 = Unbundle By Name(w1036) -> ("X"=w1028:dbl)
            n476 = Format Into String(format string="%s-%s-%s-%f-", w1029, w1026, w1027, w1028) -> (resulting string=w1038:string)  [unwired: 2 in, 1 out]
            n477 = call <userlib>:"Read XY Graph ref.vi"("error in (no error)"=w1032, "graph_utilities in"=w1033) -> ("error out"=w1041:errorcluster, "XY Graph"=w1040:refnum<vi>)  [unwired: 6 in, 2 out]
            n478 = Build Path(base path=w1030, name or relative path=w1038) -> (appended path=w1031:path)
            n479 = call <userlib>:"XY Graph to Igor Graph.vi"("error in (no error)"=w1041, "XY Graph Reference"=w1040, "Path"=w1031) -> ("error out"=w1039:errorcluster)  [unwired: 7 in, 1 out]
          }
          frame "Intensity 2" {
            n480 = local read "Intensity 2"() -> (w1047:T6)
            n481 = Format Into String(format string="%s-%s-%s-", w1046, w1047, w1043) -> (resulting string=w1049:string)  [unwired: 2 in, 1 out]
            n482 = Unbundle By Name(w1055) -> ("Intensity 2"=w1052:refnum<class "graph_utilities.lvclass">)
            n483 = Build Path(base path=w1045, name or relative path=w1049) -> (appended path=w1044:path)
            n484 = call <userlib>:"Read Intensity Graph ref.vi"("error in (no error)"=w1051, "graph_utilities in"=w1052) -> ("error out"=w1053:errorcluster, "Intensity Graph"=w1054:refnum<vi>)  [unwired: 6 in, 2 out]
            n485 = call <userlib>:"Intensity Graph to Igor Graph.vi"("error in (no error)"=w1053, "Intensity Graph Reference"=w1054, "Path"=w1044) -> ("error out"=w1050:errorcluster)  [unwired: 7 in, 1 out]
          }
          frame "H Cut 2" {
            n486 = local read "Intensity 2"() -> (w1063:T6)
            n487 = Unbundle By Name(w1072) -> ("H 2"=w1060:refnum<class "graph_utilities.lvclass">)
            n488 = call <userlib>:"Get Intensity Graph Cursor (Control).vi"("error in (no error)"=w1058, "graph_utilities in"=w1060) -> ("error out"=w1057:errorcluster, "Cursor.Cursor Position"=w1061:T19, "graph_utilities out"=w1059:refnum<class "graph_utilities.lvclass">)  [unwired: 7 in]
            n489 = Unbundle By Name(w1061) -> ("Y"=w1056:dbl)
            n490 = Format Into String(format string="%s-%s-%s-%f-", w1064, w1063, w1062, w1056) -> (resulting string=w1067:string)  [unwired: 2 in, 1 out]
            n491 = call <userlib>:"Read XY Graph ref.vi"("error in (no error)"=w1057, "graph_utilities in"=w1059) -> ("error out"=w1071:errorcluster, "XY Graph"=w1070:refnum<vi>)  [unwired: 6 in, 2 out]
            n492 = Build Path(base path=w1068, name or relative path=w1067) -> (appended path=w1065:path)
            n493 = call <userlib>:"XY Graph to Igor Graph.vi"("error in (no error)"=w1071, "XY Graph Reference"=w1070, "Path"=w1065) -> ("error out"=w1069:errorcluster)  [unwired: 7 in, 1 out]
          }
          frame "V Cut 2" {
            n494 = local read "Intensity 2"() -> (w1082:T6)
            n495 = Unbundle By Name(w1089) -> ("V 2"=w1077:refnum<class "graph_utilities.lvclass">)
            n496 = call <userlib>:"Get Intensity Graph Cursor (Control).vi"("error in (no error)"=w1074, "graph_utilities in"=w1077) -> ("error out"=w1075:errorcluster, "Cursor.Cursor Position"=w1078:T19, "graph_utilities out"=w1076:refnum<class "graph_utilities.lvclass">)  [unwired: 7 in]
            n497 = Unbundle By Name(w1078) -> ("X"=w1073:dbl)
            n498 = Format Into String(format string="%s-%s-%s-%f-", w1083, w1082, w1081, w1073) -> (resulting string=w1085:string)  [unwired: 2 in, 1 out]
            n499 = call <userlib>:"Read XY Graph ref.vi"("error in (no error)"=w1075, "graph_utilities in"=w1076) -> ("error out"=w1088:errorcluster, "XY Graph"=w1087:refnum<vi>)  [unwired: 6 in, 2 out]
            n500 = Build Path(base path=w1080, name or relative path=w1085) -> (appended path=w1079:path)
            n501 = call <userlib>:"XY Graph to Igor Graph.vi"("error in (no error)"=w1088, "XY Graph Reference"=w1087, "Path"=w1079) -> ("error out"=w1086:errorcluster)  [unwired: 7 in, 1 out]
          }
        }
        n502 = call <vilib>:"Add State(s) to Queue__jki_lib_state_machine.vi"("State(s) in (\"\")"=w995) -> ("States Out"=w994:string)  [unwired: 14 in]
      }
    }
  }
